vi "PECT - Scan no trigger.vi"() -> ()   [LabVIEW 2018]
uses:
  <vilib>/DAQmx/write.llb/DAQmx Write (Analog 1D Wfm NChan NSamp).vi
  <vilib>/DAQmx/read.llb/DAQmx Read (Analog 1D DBL 1Chan NSamp).vi
  <vilib>/DAQmx/read.llb/DAQmx Read (Analog Wfm 1Chan NSamp).vi
  <vilib>/DAQmx/create/channels.llb/DAQmx Create Channel (AI-Voltage-Basic).vi
  <vilib>/DAQmx/configure/timing.llb/DAQmx Timing (Sample Clock).vi
  <vilib>/DAQmx/configure/task.llb/DAQmx Configure Logging (TDMS).vi
  <vilib>/DAQmx/configure/trigger.llb/DAQmx Start Trigger (Digital Edge).vi
  <vilib>/DAQmx/create/channels.llb/DAQmx Create Channel (AO-Voltage-Basic).vi
  <vilib>/DAQmx/miscellaneous.llb/DAQmx Fill In Error Info.vi
  <vilib>/Instr/_visa.llb/VISA Configure Serial Port (Instr).vi
  <vilib>/express/express analysis/Spectral/Block/exnSpectralBlock spectral measurements PSD poly.vi
  <vilib>/express/express analysis/Spectral/Block/exnSpectralBlock spectral measurements PSD WFM.vi
  <vilib>/express/express analysis/Spectral/XNode/ExpressSpectralMeasurementsBlockNode.xnode
  <resource>/objmgr/daqmx.rc
  <vilib>/measure/NI_MABase.lvlib
  <vilib>/Platform/NI_3dgraph.lvlib
  <vilib>/DAQmx/read.llb/DAQmx Read (Counter U32 1Chan 1Samp).vi
  <vilib>/DAQmx/create/channels.llb/DAQmx Create Channel (CI-Count Edges).vi
panel:
  out "숫자형 2":i32
  out "숫자형 3":i32
  in  "Stop Scan 2":bool
  in  "Scan 2":bool caption="Scan"
  in  "Move Distance (mm)":dbl=16.64
  in  "Counter":tag="Dev1/ctr0"
  in  "ViewMode Analysis":i32(ring) items=["cwViewXYPlane", "cwViewXZPlane", "cwViewYZPlane", "cwViewUserDefined"]
  in  "Plot style Analysis":i32(ring)=5 items=["cwLine"=1, "cwPoint"=2, "cwLinePoint"=3, "cwHiddenLine"=4, "cwSurface"=5, "cwSurfaceLine"=6, "cwSurfaceNormal"=7, "cwContourLine"=8, "cwSurfaceContour"=9]
  in  "Open":bool
  in  "Save Scan mode":bool caption="Save Process"
  in  "Tab Control 2":T1(tab)
  out "Hall sensors signal":waveform(dbl)[](graph)=[{"t0"=timestamp(3525645621.636764 s since 1904-01-01), "dt"=1.9999999999999944e-06, "Y"=array[2100 elements], "attributes"=variant("NI_ChannelName"=variant(string "Dev1/ai0"), "NI_UnitDescription"=variant(string "Volts"))}, {"t0"=timestamp(3525645621.636764 s since 1904-01-01), "dt"=1.9999999999999944e-06, "Y"=array[2100 elements], "attributes"=variant("NI_ChannelName"=variant(string "Dev1/ai0"), "NI_UnitDescription"=variant(string "Volts"))}]
  out "Feature Extraction":dbl(graph)=0.021153968958947764
  out "Waveform Graph 2":waveform(dbl)[](graph)=[{"t0"=timestamp(0 s since 1904-01-01), "dt"=1.25e-06, "Y"=array[8000 elements]}]
  out "Power spectral density":cluster{"f0":dbl, "df":dbl, "magnitude":dbl[]}[](graph)=[{"f0"=0.0, "df"=238.09523809523876, "magnitude"=[-25.4340272409559, -28.495970805276507, -69.09064054555873, -79.11355871279994, -75.69366097931027, -84.18131507822396, -80.50168881348966, -82.72314293089615, -87.19630499623688, -82.83568021481967, -89.95290866002237, -85.90392585035596, -87.41269111550386, -91.40893948681482, -86.69370819914215, -93.36336146616782, -89.019380476413, -89.73232030153878, -94.58261196624535, -89.16287927388944, -94.965890302584, -91.86846413178648, -91.95327957161693, -97.62687167891286, -91.59993648735762, -97.30685711015555, -93.8350762480425, -93.27921214218685, -99.59438563802183, -93.1824258709588, -98.3113125531512, -95.45425138584356, -94.39327135467576, -100.65352961491782, -94.55889081970952, -99.40788907105079, -97.93617495318924, -96.19517579047603, -103.97036797797732, -96.40295202889732, -99.7036956909043, -99.48760137175819, -97.46192979187015, -106.29271483151813, -97.51447379981207, -99.86179280251669, -100.43811038443037, -97.59011642740829, -105.58363666166275, -99.01126121197593, -101.01575323613292, -101.90167607549864, -98.61952569586691, -106.73670466995647, -99.29976101634999, -101.54959604687718, -105.17330050767885, -100.09392305285375, -109.78264848704497, -100.98914236173123, -101.81665207962125, -105.42358374403365, -99.82880728595141, -107.07330885402075, -101.07712607444097, -101.03780825357597, -107.32811151840846, -101.221643458408, -105.63776326231454, -101.8420593566944, -101.80081629073969, -107.47915505307212, -101.12986632760553, -106.84901404755908, -102.73715610491038, -101.51552854007832, -107.28771371003282, -101.3928633472346, -107.44515355816633, -104.89304864643535, -103.1455098860718, -110.19910428997925, -102.73063833081197, -107.57101838377707, -104.90574568581201, -103.72599931018533, -109.97178587260123, -103.24611921258705, -108.36098023558972, -106.6408311450923, -104.73569536588386, -116.21683530762306, -105.02627439976544, -107.15856030450797, -109.81191038702062, -105.53476822084077, -119.10077766590356, -105.31867536160968, -106.9718410299748, -108.34458911268797, -104.70307996109247, -114.76704583683203, -106.29948298493936, -108.55077108437321, -112.16618350190343, -105.98453547558171, -114.68576835450673, -107.50968901677987, -107.89174277914348, -111.59875709602721, -106.69368240333122, -114.93273233954758, -105.23904516482949, -106.00272331017348, -110.36103151258544, -104.93177986717492, -110.8835476773746, -106.69346348818806, -106.66103973993782, -119.11729839814336, -108.06338160849775, -114.5879267769655, -108.59816838472844, -107.53189260743514, -114.07390818184973, -106.70996756049796, -113.27381274118753, -109.50270539577696, -107.37282420343303, -113.4779718725949, -106.04267666963091, -111.30294425571472, -112.46717993668915, -109.13164915488709, -116.65287200885172, -107.03002573045511, -110.21479040603631, -112.476075561056, -106.97710947409149, -119.42145279296255, -108.3200486628316, -110.46641858585929, -117.16650627564961, -109.73297826697552, -120.31689830731365, -107.19513745371916, -110.66663569403087, -113.30365980039964, -110.01971553524372, -123.68660617105166, -110.8171755739396, -111.11382172813546, -117.76239209582961, -109.49899370205401, -115.22252846498625, -111.1932077339224, -112.38235939086871, -118.22207022901702, -110.6546796895719, -116.97450780644367, -110.82401674194465, -111.96705198878843, -118.28092956599232, -110.5621503678909, -121.25720613496851, -111.98371482341479, -113.27928013246557, -111.96833712758355, -108.56859286664552, -120.32790468431601, -110.82699792221703, -110.79062667340345, -122.65756767769517, -110.48843456045427, -116.8782055296399, -115.43719816168479, -114.47619780315773, -121.42183196132746, -111.60631415727042, -120.68077308056417, -109.35478690141552, -109.03210709352732, -120.6260555904793, -109.47936424950136, -113.33719701518146, -112.88325992990137, -110.99901978536154, -123.19636626521421, -109.09861317900774, -113.33125158106256, -115.35673297389727, -112.77249677632989, -124.61163141716472, -114.68140920359865, -121.89642913325117, -115.47413298424323, -112.82196063671608, -127.87542521315149, -111.54178118788309, -113.6448752704395, -120.76569423868874, -112.98651214877823, -123.18868565400437, -115.41399838634062, -115.46853076016815, -116.40989072804102, -110.69611347288615, -132.23164080331392, -114.76376391429793, -121.7246597336247, -117.46893009589195, -114.01899156779395, -125.22079066032327, -114.59524199183258, -114.50034890537415, -122.9532092227648, -113.72727798159212, -125.65163915514907, -113.4793801211504, -110.4090756414644, -125.63592649005872, -114.22938378193007, -116.74947251106808, -121.60535557984142, -116.79385283402802, -122.44667696630361, -113.43873413563811, -123.28159708694415, -113.92892974938164, -114.01193823589753, -121.62751955742443, -118.76839573694522, -125.52998605097204, -115.19609643487229, -117.49409595176479, -117.08423885198002, -119.48314867245172, -125.01675515413412, -117.92668164142911, -115.55962389856793, -125.63488616674975, -119.11862859365166, -114.78860770332909, -117.18339781294443, -111.18063004722558, -118.31775966044624, -111.6867367949252, -114.57226159377, -119.36541212960576, -113.90245139442648, -132.46343443313128, -120.1282759002165, -121.05279009698619, -118.9115822659523, -121.23280439248342, -116.31914159559688, -127.38829313950257, -117.34673005740623, -115.95249861902771, -114.9301657394146, -123.22361802797445, -110.83274939062106, -116.16624248562111, -116.76753364192771, -113.94454545069023, -122.95736945775944, -118.66755800656253, -129.1462641201204, -116.6351050110328, -117.22529407303742, -123.80212197360244, -115.89792176423389, -114.25823938606595, -125.60467961977515, -114.59958849364433, -121.70071005514421, -118.25968972451209, -114.69929400946009, -123.88209034116528, -115.03869272537257, -117.52034211782204, -115.27990843516797, -117.85366603932033, -125.16865559622727, -118.21960424638507, -119.69008755413566, -117.24640963460672, -114.32867295013791, -119.1576982419508, -122.85495988425586, -116.3373010103401, -114.53730203699834, -115.67017599990201, -127.144321037601, -115.73849102686786, -117.7626163106355, -119.7346592991025, -117.41317517684553, -125.0417974461613, -114.5488949833583, -116.59812516173781, -119.91064563147799, -115.27933218667663, -122.09990513751134, -120.95678574143693, -123.25641714743752, -112.5173710452192, -113.53735878806998, -129.23914933506734, -116.27157269711533, -148.4020512032711, -118.84888216023774, -123.82550527215588, -116.87770979616658, -111.32191810025745, -124.32675905891588, -114.37182733794062, -121.10713785851372, -122.59698730059695, -116.38346694563282, -121.69144349152856, -119.00883142493832, -110.81886738196273, -120.7909830607913, -115.01780448665316, -114.52055121633796, -132.6824191654361, -116.330695115645, -126.4664151018508, -118.32717907779282, -118.7288071595281, -120.42749846140066, -112.53185615773879, -124.26026008984286, -114.24089252048742, -120.00368190003405, -114.71738500842926, -112.92262025927133, -129.21127897188563, -113.5947811765517, -117.80802009651353, -117.0133790103226, -112.19210322760304, -118.17549968071762, -119.3256187825503, -118.84981507334446, -121.39118969751144, -114.64543555194373, -119.84814933224528, -114.09123407848944, -116.22899352170892, -116.41650104077173, -113.70057202673476, -124.52773908304957, -114.87372641784933, -116.11651108221098, -121.68680962246994, -115.78306007961302, -122.22621008657796, -118.81157995182392, -113.9402115821658, -132.636729517989, -114.49554876936634, -119.50980190398928, -123.27410972236837, -118.52851881066383, -122.25212982572599, -117.13947036230024, -120.85005588797962, -118.41526503460501, -117.61788553858068, -126.3872056783977, -114.98198608543298, -119.7789938911847, -120.84873579392627, -114.38831474301695, -153.35954756825245, -113.19505610638078, -114.17454820985151, -127.41069917723112, -114.92677241657191, -125.49053973810628, -113.36382196587914, -119.96785250843519, -122.47388530423243, -116.38671253508838, -120.0905790211523, -119.83326265062107, -117.88168146696918, -122.3132169880757, -115.87324909105399, -125.92003267803432, -113.96860176867415, -114.49156118371398, -127.52634390035722, -115.05967156528004, -126.82020221981517, -117.93643187259194, -116.51163213641807, -119.47551219110167, -119.55225172256931, -116.9512257852571, -122.23153124485954, -120.8368476753637, -121.48473913072222, -115.83122660909913, -135.74260014140523, -116.58358375805423, -118.15236945484727, -119.06674062398864, -115.7844834762477, -125.06111738611818, -114.7801535050972, -115.2696605691888, -123.98656374010793, -119.29025555731172, -118.29146803784099, -119.55696172158135, -118.06884171238352, -127.81587648134607, -120.41730580797976, -123.49626136731604, -112.2147141798107, -116.22555232584983, -132.79419178871254, -119.66964883124663, -117.20946469243259, -118.20939292735417, -115.6951914646649, -129.64892855822356, -114.27056999288617, -120.31005512957381, -117.41846777372632, -115.50158386260813, -124.69777160737624, -115.2892897247205, -123.61522771666871, -113.75248734362687, -113.22999749252833, -129.3490509395313, -116.88137735661701, -116.94110280242681, -119.50244079984806, -119.30521139999144, -128.17199984115797, -118.06736594940236, -116.05331575995922, -121.29670750650897, -116.1140297602044, -125.090619084802, -121.41807296062154, -120.01332757902264, -120.54914530643151, -116.49738633175463, -122.32551291835904, -118.3190808346865, -118.92638453656723, -122.48819531011718, -117.01021725424317, -120.98896352560598, -117.23831688685218, -121.27915259197124, -121.20017251921661, -117.6155648860373, -120.91300272912063, -117.94438460863424, -115.94437430101533, -123.35904829443987, -117.74011174503076, -121.54935745388448, -120.82564553545025, -121.98951430455743, -120.24858103448778, -116.44403527138395, -112.79571494351876, -112.42801913096545, -110.1697573019791, -115.34500457736401, -119.81921052956707, -129.82600951154313, -115.5862301263047, -112.59292882433087, -120.79009137478283, -131.32849293387295, -113.61194478398238, -123.48568856527031, -119.17507777781304, -123.09261867490484, -116.97755217417308, -123.94453461434183, -116.58080525616379, -119.64289646280756, -122.90202645580743, -126.66219093058154, -121.95048829056148, -115.72578023509817, -116.70117814464484, -121.91050280869723, -118.25299095698178, -116.45905559047064, -132.57794493731578, -121.65327820443292, -120.9816664775787, -117.17270262269045, -120.27433984830965, -125.89418976028173, -119.09563505847817, -126.9693215534833, -113.17465524665704, -118.98702092883116, -119.83822568580342, -120.45832738089722, -120.67735960513633, -127.38676010839353, -127.65777338183055, -118.37446329057411, -115.61355494839711, -119.94568688114103, -116.06619937633681, -126.348857777089, -118.92850079147068, -119.5416617639739, -132.47075644221843, -118.08809356028496, -123.16186463092723, -121.51579486791232, -122.88983670053283, -129.5195538417256, -120.4730389608841, -132.16486858341602, -122.34690358436781, -120.71922104337597, -114.29260860841114, -117.67902631803368, -124.7040155514909, -123.51274592117205, -120.02297921674332, -136.54655493811157, -120.45629227407751, -119.06410204276258, -127.91681714792554, -122.82090055753153, -125.16838176650813, -121.79565386970478, -119.79607311590995, -126.54861375039647, -121.59135878113302, -132.8348640697562, -118.1305434733294, -120.46070148841905, -122.69571910896963, -117.6534954653865, -124.15742546824006, -120.73646926947502, -124.82696993800742, -124.513836786494, -123.15395713389651, -124.62395468806395, -117.21365768658171, -119.32635871968456, -121.48532284413152, -119.38242892643675, -126.25575652510352, -123.27133124029851, -117.58533922728374, -118.17710108929799, -114.99496360200965, -117.77133194647278, -111.34898201101595, -111.50817058307922, -119.0703124690998, -127.70676079885351, -121.8704969141074, -125.93154214283446, -118.65628450081473, -122.47918878348962, -117.9651589546518, -126.13560583004508, -122.42294805637847, -133.924453763793, -117.2082573038767, -117.6525335446734, -122.92077297426977, -122.04624645756786, -116.43289028226238, -117.93180959338378, -129.02356734231915, -117.95493621286326, -120.7555929766252, -120.76782849311112, -123.06287498470708, -117.83798593857965, -123.43423215434719, -120.15190119516652, -120.48240443128407, -143.29738987393452, -123.46572247444769, -120.89055325172792, -125.66715973809033, -118.26887578998644, -117.01836200028421, -121.33021830755509, -119.68846363313813, -122.60689066103069, -116.26858138914181, -119.59360791972998, -122.94866175463353, -114.174409515556, -118.00516930888391, -121.56978543579633, -135.87799017759036, -117.50816594504829, -122.82539428457626, -123.82103443155845, -124.77975840345442, -121.13340798086698, -120.93607435603558, -133.15787160745222, -120.70545628137863, -125.02155972441679, -122.04666465472178, -118.01234649746348, -127.88767491042842, -119.02096620167217, -120.16031065152875, -122.25406107859625, -121.72733059051095, -120.61357375519918, -118.63962847172827, -134.3857741605498, -116.3600853185034, -117.26695700691671, -119.9176982185873, -113.45576465218444, -126.69779573632724, -114.39554522802246, -116.8457146515868, -116.34219889483086, -119.30011291548334, -120.01163291843496, -114.29497178248809, -127.65687642749229, -119.58556923753022, -129.8593054181261, -122.2353645100479, -120.79536520223796, -119.83284028355028, -117.7991246185715, -128.390292904734, -119.78079925213122, -125.478913448993, -113.89747777944768, -112.66620124153357, -124.3475049842711, -120.85847303094337, -132.91807981902295, -119.523494985723, -116.65149909866443, -119.73287290436721, -127.63237851524192, -127.23413304048789, -120.87585453904362, -121.08540368080186, -134.91071939669257, -117.75375801669338, -117.2683014590723, -120.9739099492833, -118.23809733632451, -120.94065804928206, -123.88077510875804, -118.13812819300607, -122.60294123365466, -126.97075898006995, -120.18754789731035, -124.71238663441227, -120.55456557278582, -130.94599087480253, -111.18288669417035, -112.27708791831247, -126.0512034600378, -117.41881712783596, -128.20553880273903, -117.29482600885808, -118.2045526390752, -127.81966672699878, -117.03716165902529, -115.46711739757512, -117.15363929234843, -121.87599671671335, -121.19736800869221, -126.5301786755875, -131.20754947382918, -124.40138004810741, -129.0562496906515, -121.06816554587536, -121.01023627802867, -138.6137911215848, -120.12495002524031, -121.38510517514229, -122.79804220535513, -116.97501378195477, -118.82011581137473, -114.0229185604644, -119.54287501990726, -114.64474566771625, -117.76935669872461, -123.81082574158907, -118.51678358865587, -128.9664755188374, -123.45357998434133, -122.74888841574231, -120.74640581234044, -126.956344345126, -119.95682140104577, -118.8873101779055, -124.41062359284174, -128.97304498664363, -123.86287113204068, -127.30257087528216, -120.61364220528216, -114.45119129304715, -119.68384044686806, -131.29639185291157, -122.31250766293485, -119.57420865241102, -124.74014026002448, -124.87593035709094, -118.4566565612952, -123.76236085976001, -120.84780538841838, -117.68987599773281, -135.06195695255914, -122.56143585795171, -129.04610316842883, -118.32313199570537, -117.77093802786419, -124.46572845786741, -129.1123298336903, -120.88470269965448, -116.69988985752187, -116.84054667499878, -133.76883696987278, -122.32434984927302, -124.98940594457933, -122.56515592789917, -118.31562562243366, -133.97049179545627, -122.33220627999802, -131.16753675316977, -124.69828063969263, -116.37621154460467, -126.1833423168025, -129.62937634161355, -118.46241371150788, -117.52851478852457, -125.32425037236442, -119.0327364293772, -124.2861355894013, -123.24573502278234, -125.52155812053758, -113.75743410709823, -114.79513162658353, -128.58142362588052, -122.48277095196701, -118.94747544412269, -123.86988127835491, -124.78140456983323, -121.53998481875398, -116.01432822539552, -119.20174681160661, -122.75167725800814, -120.58657749420254, -118.51141061842183, -119.24457006171983, -131.43641234223372, -116.00759139055087, -121.24442216102587, -123.29371279953725, -117.608355420454, -116.33684374617326, -118.06291688281922, -121.88761866022774, -121.54820313120047, -119.5051369873635, -126.56611158390913, -118.84012713615805, -121.09285296522563, -124.67955377692547, -147.31451139022337, -116.80660421066897, -114.8367853755961, -120.41026468628925, -123.65666101895222, -119.64837119787269, -116.77480172559095, -116.54263359173909, -124.75286620868079, -117.33721912698883, -116.51795620907136, -118.50086748176733, -128.10381328920522, -122.78098994574157, -120.24716756092855, -119.52743204722819, -115.00407387659232, -108.2853711552629, -108.61086943894702, -119.6228894146785, -124.11132022420912, -125.6202218409766, -123.1749360787656, -118.1971196161698, -123.95075368058998, -121.72140109898365, -123.27106899042522, -123.73035629887062, -121.24369679109273, -121.07381526465288, -113.13965659723667, -118.330755475899, -118.40249076804484, -111.59630598649044, -116.1569506845575, -125.67326089915758, -125.85723567111906, -119.24293277595024, -117.87067617433537, -120.70936924059559, -131.8090588468898, -132.98711569625004, -123.63274249467587, -122.75476917502559, -126.12873814250243, -120.53144270605179, -129.07030822919336, -122.7889410422919, -124.35405971166259, -119.63968579420454, -139.0154441054289, -129.47962001806934, -121.86548015410847, -128.6818469257012, -121.40195873232601, -138.64231053781285, -124.22025721762265, -124.06073958736941, -126.71929802352521, -131.7498459276443, -120.68144109742178, -122.6325588818875, -126.80796617875095, -124.92487955227033, -136.94498040498806, -124.26704334219014, -123.21376211221711, -140.25352033075964, -129.53222319772195, -122.58541579060463, -122.1996729592375, -125.66642108013673, -125.66310429236694, -120.09682773706965, -125.27326633941439, -121.55721878725502, -121.22507119941083, -121.53716878624485, -136.20685498111987, -128.15260146013156, -120.03473972471616, -124.60755958763912, -124.73082500077143, -123.93425949983688, -131.04483249265184, -121.7957035014449, -127.09321441816094, -133.6144579272493, -124.69014595896968, -130.4902091211609, -121.18031440773905, -128.00033943961677, -125.88991118115149, -118.865310745079, -123.69668867733147, -117.98756965862728, -114.40013091842827, -118.28685032521078, -122.23464196869948, -124.8440422629961, -129.66281606870848, -119.440534215621, -124.54391783563877, -124.93447967158188, -121.7258558761523, -122.28817885403082, -127.06889620458577, -128.92172974939206, -120.62932166634072, -126.06847321900452, -123.31471168429935, -121.80350826545656, -129.2574604322076, -125.67225933193998, -125.7801671825605, -129.53804733161627, -119.56756644124712, -128.82490314699373, -124.7689736295626, -120.50019729114693, -124.50603158563972, -122.8120627011088, -125.60528875555717, -123.8817354922713, -124.05570537836674, -120.94568834491936, -118.06056028605255, -124.24390361274648, -125.5716703018188, -127.71949519914061, -130.7001652968252, -126.27701412017494, -133.76810134709916, -128.4738939614179, -120.302550881701, -118.91298143662928, -124.9077318110765, -127.16253699189492, -118.11405934812818, -117.52028071290711, -140.95620572748925, -123.61977932545628, -131.0334379970501, -125.88948384968432, -127.81552331993379, -121.92316280719056, -119.05911238768732, -126.83773251459189, -123.52627415002164, -120.8779561023192, -123.66683567603742, -131.64300993967345, -123.62895847772963, -116.89792951363142, -120.1068259250195, -117.92484706459337, -115.58208487778379, -120.76803581628594, -123.95408562090736, -122.79456549632754, -134.5305398779298, -123.57040300991032, -128.40634159414552, -123.70102187824159, -118.24970739397313, -119.66483900349026, -127.78024313111393, -120.3547204111785, -125.49305364308705, -119.49505591004302, -120.50920386196539, -119.03509516851003, -114.24667300009652, -121.60538636584391, -119.95304417598024, -122.24585853682832, -128.63653016912684, -116.04810628805795, -121.94159862131235, -122.59928204398939, -121.4532410501923, -128.6511474663462, -130.83715595958148, -121.71998300574741, -116.91426629511156, -113.587592058512, -115.59736707638731, -124.65300822631244, -133.32538684258748, -124.02289142873636, -121.54278890993639, -119.02596809402394, -108.90572887117857, -112.14974069608851, -129.21149299565423, -118.82148342951197, -116.65510894288538, -118.39609618084175, -116.53502642884725, -122.47549439965209, -122.23125657046063, -123.68081343116663, -120.67915071600007, -123.6899360128769, -118.56721985209728, -118.36641581191942, -126.96724630704657, -119.36877661672403, -123.07698921198843, -117.80772421906035, -122.82545076270567, -118.82755071380888, -117.21030132539394, -129.760567864525, -118.0816708063509, -125.80573274113647, -121.18434666182338, -121.80987210832065, -130.99259828357094, -125.47223579895922, -123.86818606677002, -118.7118158196511, -119.27778317338742, -127.27333258839096, -119.90672352079164, -140.78772370844268, -118.08251080057329, -119.86636232122572, -118.69482489738232, -119.19106512767372, -123.70988914879189, -121.92566832147995, -123.41378261726373, -120.1715186070818, -117.9079629421116, -117.41960207545632, -123.72833996166874, -127.24377206607298, -124.99098647980887, -129.48803701799955, -129.92351350561592, -120.79284154834647, -119.29601975194524, -136.17244775530037, -126.73975437546255, -128.84068276143336, -125.66374985701982, -136.69026010435715, -125.44409235146617, -119.28138070315057, -118.65017329869724, -118.02521532826772, -122.23736063759657, -121.27846943548622, -116.69850478126861, -119.7711336696722, -123.70776561180185, -118.43344549561263, -123.92390877157247, -117.19637143066551, -117.64112988205311, -127.78399195238529]}, ...(2 in all)]
  in  "3D Surface":refnum<k7>(container)
  out "Feature Extraction 2":dbl(graph)=0.021153968958947764
  in  "Emergency Stop":bool
  in  "Stop 3":bool
  in  "Home Y":bool
  in  "Home X":bool
  in  "Back":bool
  in  "Front":bool
  in  "Left":bool
  in  "Right":bool
  in  "Stop Scan":bool
  in  "Scan":bool
  in  "Tab Control":enum32{"     Motor    ", "         DAQ        "}(tab)
  out "Y line":i32 caption="Y percent"
  in  "Move X":bool
  in  "X-length":dbl=20.0
  in  "Y-length":dbl=20.0
  in  "Step Y":dbl=0.2
  in  "1 Min":dbl=0.4
  in  "2 Max":dbl=6.0
  in  "1  Max":dbl=6.0
  in  "2 Min":dbl=0.4
  in  "1 Rate":dbl=0.2
  in  "2 Rate":dbl=0.4
  in  "Travel per Pulse (mm)":dbl=0.002
  in  "Cur. Pos X":dbl=-33.28 format="%#.4f"
  in  "Cur. Pos Y":dbl=30.0 format="%#.4f"
  in  "Save Speed":bool
  in  "COM Port":refnum<visa-resource-name>="COM4"
  in  "Baud Rate":u32=9600
  in  "Data bits":u16=8 min=5 max=8 step=1
  in  "stop bits":u16(ring)=10 items=["1.0"=10, "1.5"=15, "2.0"=20]
  in  "Parity":u16(ring) items=["None", "Odd", "Even", "Mark", "Space"]
  in  "Logging Mode":i32(ring)=10231 items=["Off"=10231, "Log and Read"=15842]
  out "Actual Sample Rate":dbl=500000.0 format="%0.2f"
  in  "Physical Channel":tag="Dev4/ai0"
  in  "Min Voltage":dbl=-10.0
  in  "Max Voltage":dbl=10.0
  in  "Terminal Configuration":i32(ring)=10083 items=["default"=-1, "RSE"=10083, "NRSE"=10078, "Differential"=10106, "Pseudodifferential"=12529]
  in  "Sample Clock Source 2":tag="OnboardClock"
  in  "Sample Rate":dbl=500000.0
  in  "TDMS File Path":path
  in  "Number of Samples 2":i32=160
  out "Actual Sample Rate 2":dbl=800000.0 format="%0.2f"
  in  "Physical Channel(s)":tag="Dev4/ao1"
  in  "Min Voltage 2":dbl=-10.0
  in  "Max Voltage 2":dbl=10.0
  in  "Sample Clock Source":tag="OnboardClock"
  in  "Sample Rate 2":dbl=800000.0
  in  "Number of Samples":i32=8000
  in  "Offset":bool
  in  "2 Plots":bool
  in  "Edge":i32(ring)=10280 items=["Rising"=10280, "Falling"=10171]
  in  "Digital Trigger Source":tag="/Dev4/PFI0"
  in  "Average":i32=10
  in  "Duty cycle %":dbl=50.0 format="%#.2f"
  in  "Stop":bool
  in  "Output Array":T2(array[cluster])=[{"Waveform Type"=2, "Amplitude"=10.0, "Frequency"=300.0}] {"Frequency" format="%0.2p"; "Amplitude" format="%0.2p"; "Waveform Type" items=["Sine Wave", "Triangle Wave", "Square Wave", "Sawtooth Wave"]}
  # "Pulse Shape"
  # "Trigger Settings"
  # "Data Processing"
  # "Pulse"
  # "Hall Sensors Signal"
  # "Feature Extraction"
  # "Power Spectal Density"
  # "COM  Setting"
  # "Speed  Setting"
  # "Scan  Setting"
  # "Pulse  Channel"
  # "Pulse  Timming"
  # "Sensor  Channel"
  # "DAQ Timming"
  # "Logging Settings"
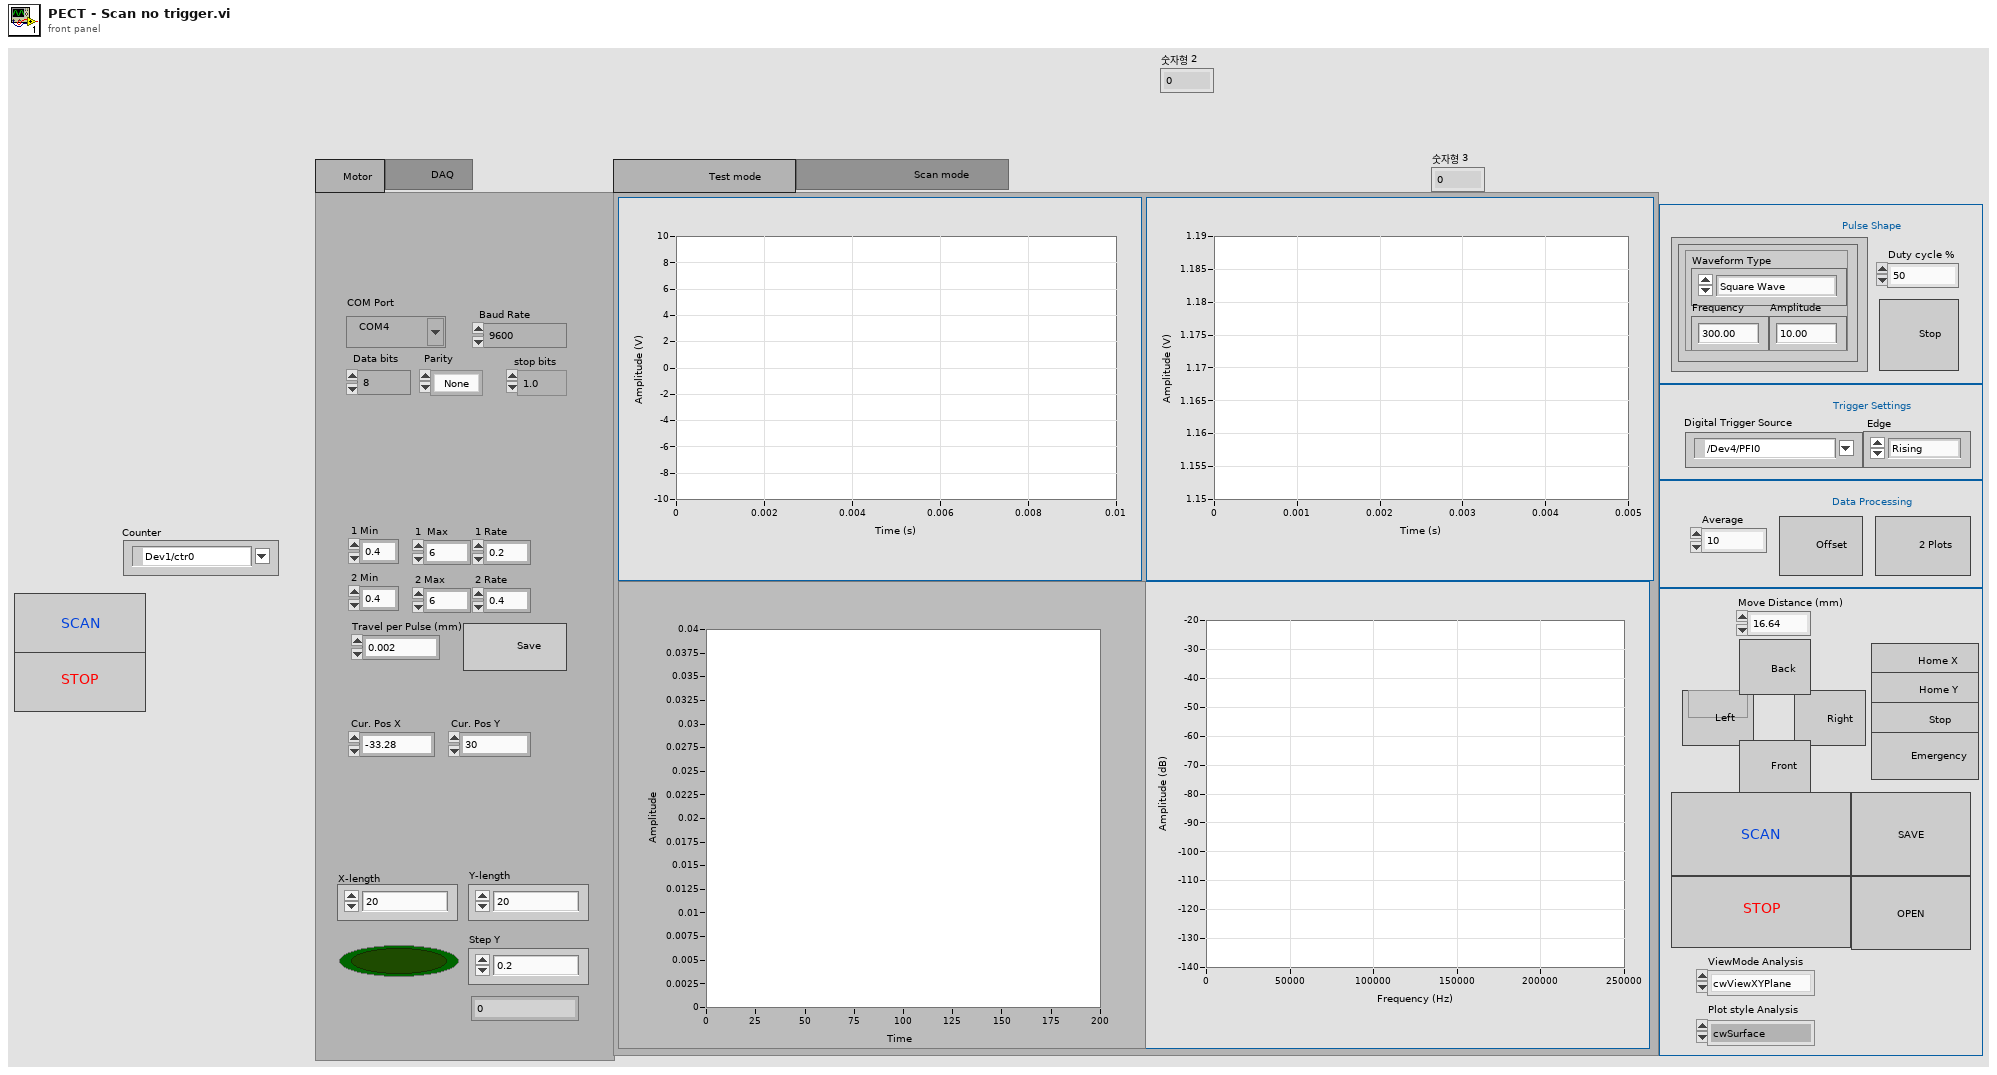
[diagram p1: front panel]
types:
  T1 = enum32{"                    Test mode                   ", "                          Scan mode                      "}
  T2 = cluster{"Waveform Type":u16, "Amplitude":dbl, "Frequency":dbl}[]
  T3 = cluster{"Waveform Type":u16, "Amplitude":dbl, "Frequency":dbl}
  T4 = cluster{"averaging mode":u16, "weighting mode":u16, "number of averages":u32}
  T5 = cluster{"dB On (F)":bool, "unwrap phase (F)":bool, "convert to degree (F)":bool}
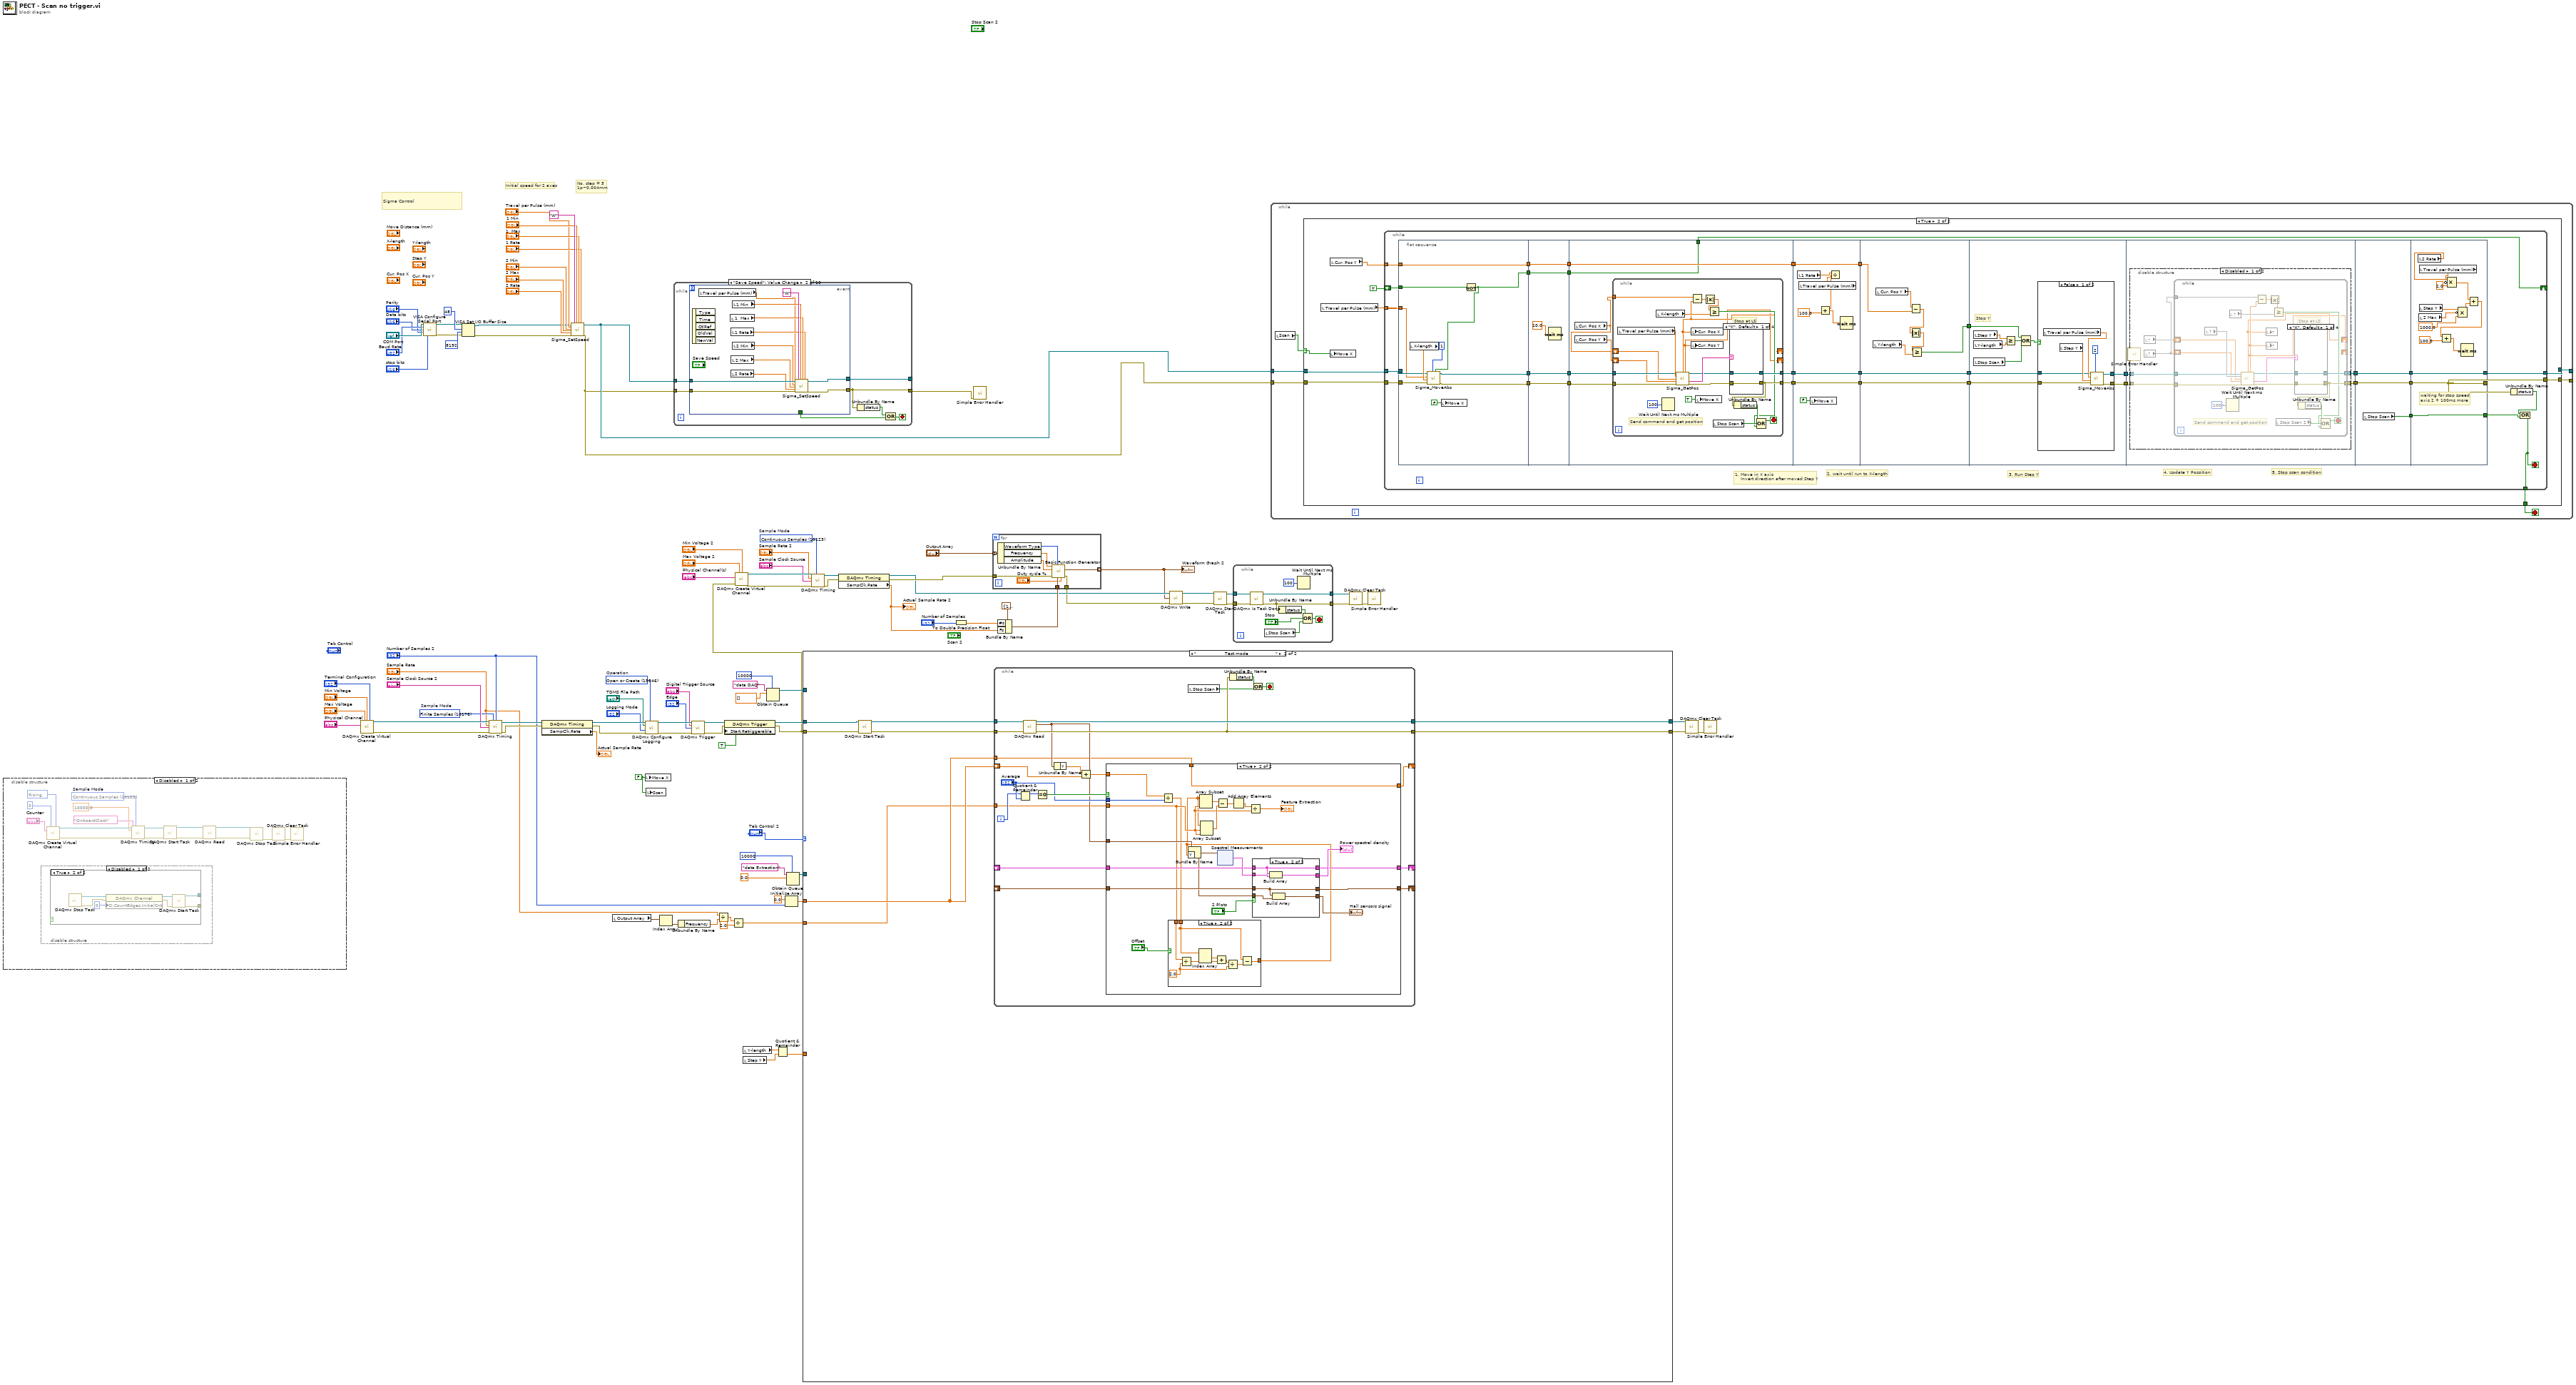
[diagram p0: block diagram]
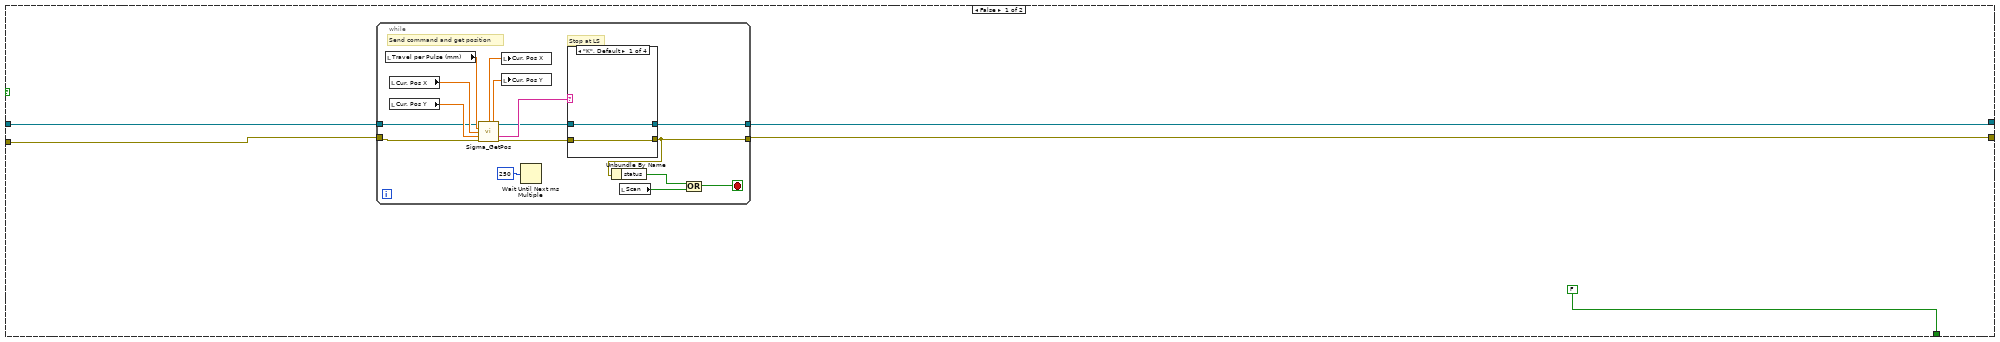
[diagram p2: hidden frame]
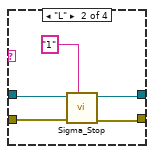
[diagram p3: hidden frame]
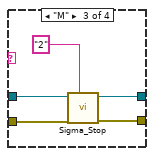
[diagram p4: hidden frame]
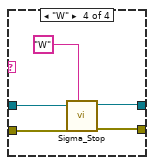
[diagram p5: hidden frame]
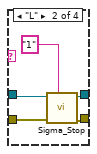
[diagram p6: hidden frame]
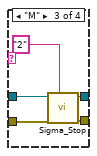
[diagram p7: hidden frame]
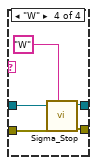
[diagram p8: hidden frame]
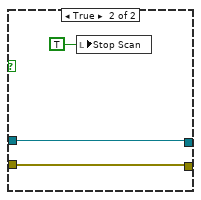
[diagram p9: hidden frame]
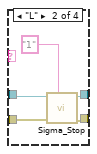
[diagram p10: hidden frame]
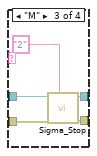
[diagram p11: hidden frame]
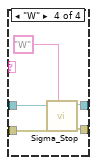
[diagram p12: hidden frame]
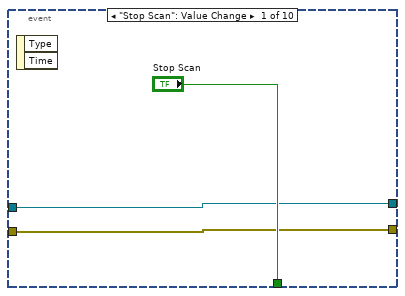
[diagram p14: hidden frame]
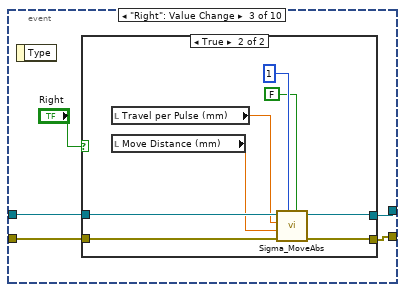
[diagram p15: hidden frame]
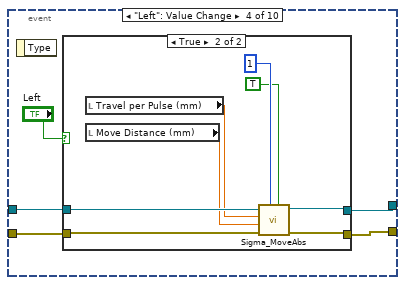
[diagram p17: hidden frame]
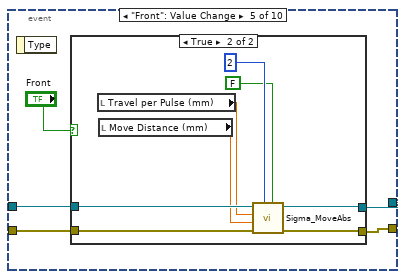
[diagram p19: hidden frame]
diagram:
  w1 = FALSE ("Move X")
  w55 = 10178 items=["Finite Samples"=10178, "Continuous Samples"=10123, "Hardware Timed Single Point"=12522]  # Sample Mode
  w78 = 10123 items=["Finite Samples"=10178, "Continuous Samples"=10123, "Hardware Timed Single Point"=12522]  # Sample Mode
  w94 = 15846 items=["Open"=10437, "Open or Create"=15846, "Create or Replace"=15847, "Create"=15848]  # Operation
  # "No. step = 5\n1p~0.004mm"
  # "Initial speed for 2 axes"
  # "Sigma Control"
  n1 = disable-structure shown="Disabled" {
    frame Disabled {
      w115 = 10280 items=["Rising"=10280, "Falling"=10171] ("edge")
      w114 = 10123 items=["Finite Samples"=10178, "Continuous Samples"=10123, "Hardware Timed Single Point"=12522]  # Sample Mode
      n2 = disable-structure shown="Disabled" {
        frame Disabled {
          n3 = case shown="True" {
            selector: _ -> [_ _]
            tunnel: [_ w120] -> _
            tunnel: [_ w117] -> _
            frame False {
            }
            frame True {
              n4 = call <vilib>:"DAQmx Stop Task.vi"() -> ("task out"=w122:refnum<k21>, "error out"=w119:errorcluster)  [unwired: 14 in]
              n5 = property class="DAQmx Channel"(reference=w122, error in=w119, "CI.CountEdges.InitialCnt"=u32 0) -> (reference out=w121:refnum<k21>, error out=w118:errorcluster)
              n6 = call <vilib>:"DAQmx Start Task.vi"("task/channels in"=w121, "error in"=w118) -> ("task out"=w120:refnum<k21>, "error out"=w117:errorcluster)  [unwired: 12 in]
            }
          }
        }
        frame Enabled {
        }
      }
      n7 = call-poly <vilib>:"DAQmx Create Virtual Channel.vi"("initial count"=u32 0, "edge"=w115, "counter"="Counter") -> ("task out"=w110:refnum<k21>, "error out"=w109:errorcluster)  [unwired: 11 in]
      n8 = call-poly <vilib>:"DAQmx Timing.vi"("task/channels in"=w110, "sample mode"=w114, "rate"=10000.0, "source"=tag "OnboardClock", "error in"=w109) -> ("task out"=w112:refnum<k21>, "error out"=w111:errorcluster)  [unwired: 9 in]
      n9 = call <vilib>:"DAQmx Start Task.vi"("task/channels in"=w112, "error in"=w111) -> ("task out"=w104:refnum<k21>, "error out"=w102:errorcluster)  [unwired: 12 in]
      n10 = call-poly <vilib>:"DAQmx Read.vi"("task/channels in"=w104, "error in"=w102) -> ("task out"=w103:refnum<k21>, "error out"=w101:errorcluster)  [unwired: 11 in, 1 out]
      n11 = call <vilib>:"DAQmx Stop Task.vi"("task/channels in"=w103, "error in"=w101) -> ("error out"=w106:errorcluster)  [unwired: 12 in, 1 out]
      n12 = call <vilib>:"DAQmx Clear Task.vi"("error in"=w106) -> ("error out"=w105:errorcluster)  [unwired: 14 in]
      n13 = call <vilib>:"Simple Error Handler.vi"("error in (no error)"=w105) -> ()  [unwired: 4 in, 5 out]
    }
    frame Enabled {
    }
  }
  n14 = call-poly <vilib>:"DAQmx Create Virtual Channel.vi"("maximum value"="Max Voltage", "minimum value"="Min Voltage", "input terminal configuration"="Terminal Configuration", "physical channels"="Physical Channel") -> ("task out"=w97:refnum<k21>, "error out"=w98:errorcluster)  [unwired: 10 in]
  n15 = call-poly "VISA Configure Serial Port"("VISA resource name"="COM Port", "baud rate (9600)"="Baud Rate", "data bits (8)"="Data bits", "parity (0:none)"="Parity", "stop bits (10: 1 bit)"="stop bits") -> ("VISA resource name out"=w12:refnum<visa-resource-name>, "error out"=w6:errorcluster)  [unwired: 9 in]
  n16 = VISA Set I/O Buffer Size(VISA resource name=w12, mask (16)=48, size (4096)=u32 8192, error in (no error)=w6) -> (VISA resource name out=w16:refnum<visa-resource-name>, error out=w15:errorcluster)
  n17 = call-poly <vilib>:"DAQmx Timing.vi"("task/channels in"=w97, "sample mode"=w55, "samples per channel"="Number of Samples 2", "rate"="Sample Rate", "source"="Sample Clock Source 2", "error in"=w98) -> ("task out"=w100:refnum<k21>, "error out"=w99:errorcluster)  [unwired: 8 in]
  n18 = property class="DAQmx Timing"(reference=w100, error in=w99) -> (reference out=w96:refnum<k21>, error out=w95:errorcluster, "SampClk.Rate"=→"Actual Sample Rate":dbl)
  n19 = call "Sigma_SetSpeed.vi"("VISA resource name"=w16, "Travel per Pulse (0.004mm)"="Travel per Pulse (mm)", "Min (1mm) 2"="2 Min", "Max (2mm) 2"="2 Max", "Rate (1mm) 2"="2 Rate", "error in (no error)"=w15, "Axis (1)"="W", "Min (1mm)"="1 Min", "Max (2mm)"="1  Max", "Rate (1mm)"="1 Rate") -> ("VISA resource name out"=w5:refnum<visa-resource-name>, "error out"=w4:errorcluster)  [unwired: 8 in]
  n20 = local read "Output Array"() -> (w45:T2)
  n21 = local write "Move X"(w1) -> ()
  n22 = call-poly <vilib>:"DAQmx Configure Logging.vi"("task/channels in"=w96, "operation"=w94, "file path"="TDMS File Path", "logging mode"="Logging Mode", "error in"=w95) -> ("task out"=w93:refnum<k21>, "error out"=w92:errorcluster)  [unwired: 9 in]
  n23 = local write "Scan"(w1) -> ()
  n24 = Index Array(array=w45) -> (element=w44:T3)  [unwired: 1 in]
  n25 = while {
    tunnel: w5 -> [w130]
    tunnel: [w125] -> _
    tunnel: w4 -> [w129]
    tunnel: [w127] -> w25
    stop <- w126 stop-if-true
    n26 = event shown="[1] \"Save Speed\": Value Change" {
      selector: _ -> [_ _ _ _ _ _ _ _ _ _]
      dyn-events: _ -> [_ _ _ _ _ _ _ _ _ _]
      timeout: _ -> [_ _ _ _ _ _ _ _ _ _]
      tunnel: w130 -> [w132 w145 w148 w163 w178 w193 w210 w222 w232 w244]
      tunnel: w129 -> [w131 w142 w147 w162 w177 w192 w209 w221 w231 w243]
      tunnel: [w132 w144 w150 w165 w180 w195 w207 w220 w234 w246] -> w125
      tunnel: [w131 w143 w149 w164 w179 w194 w206 w219 w233 w245] -> w127
      tunnel: ["Stop Scan" _ _ _ _ _ _ _ _ _] -> w124
      event "Stop Scan": Value Change {
        n27 = event-data() -> ()  [unwired: 1 in, 2 out]
      }
      event "Save Speed": Value Change {
        n28 = event-data() -> ()  [unwired: 1 in, 5 out]
        n29 = local read "Travel per Pulse (mm)"() -> (w134:dbl)
        n30 = local read "1  Max"() -> (w139:dbl)
        n31 = local read "1 Rate"() -> (w138:dbl)
        n32 = local read "2 Rate"() -> (w135:dbl)
        n33 = local read "2 Max"() -> (w136:dbl)
        n34 = local read "1 Min"() -> (w140:dbl)
        n35 = local read "2 Min"() -> (w137:dbl)
        n36 = call "Sigma_SetSpeed.vi"("VISA resource name"=w145, "Travel per Pulse (0.004mm)"=w134, "Min (1mm) 2"=w137, "Max (2mm) 2"=w136, "Rate (1mm) 2"=w135, "error in (no error)"=w142, "Axis (1)"="W", "Min (1mm)"=w140, "Max (2mm)"=w139, "Rate (1mm)"=w138) -> ("VISA resource name out"=w144:refnum<visa-resource-name>, "error out"=w143:errorcluster)  [unwired: 8 in]
      }
      event "Right": Value Change {
        n37 = event-data() -> ()  [unwired: 1 in, 1 out]
        n38 = case shown="True" "Right" {
          tunnel: [w152 w158] -> w150
          tunnel: [w151 w157] -> w149
          tunnel: w148 -> [w152 w160]
          tunnel: w147 -> [w151 w159]
          frame False {
          }
          frame True {
            n39 = local read "Travel per Pulse (mm)"() -> (w154:dbl)
            n40 = local read "Move Distance (mm)"() -> (w153:dbl)
            n41 = call "Sigma_MoveAbs.vi"("Direction (+)"=FALSE, "Axis (1)"=1, "error in (no error)"=w159, "Travel (1mm)"=w153, "Travel per Pulse (0.004mm)"=w154, "VISA resource name"=w160) -> ("error out"=w157:errorcluster, "VISA resource name out"=w158:refnum<visa-resource-name>)  [unwired: 4 in]
          }
        }
      }
      event "Left": Value Change {
        n42 = event-data() -> ()  [unwired: 1 in, 1 out]
        n43 = case shown="True" "Left" {
          tunnel: [w167 w174] -> w165
          tunnel: [w166 w173] -> w164
          tunnel: w163 -> [w167 w175]
          tunnel: w162 -> [w166 w172]
          frame False {
          }
          frame True {
            n44 = local read "Travel per Pulse (mm)"() -> (w169:dbl)
            n45 = local read "Move Distance (mm)"() -> (w168:dbl)
            n46 = call "Sigma_MoveAbs.vi"("Direction (+)"=TRUE, "Axis (1)"=1, "error in (no error)"=w172, "Travel (1mm)"=w168, "Travel per Pulse (0.004mm)"=w169, "VISA resource name"=w175) -> ("error out"=w173:errorcluster, "VISA resource name out"=w174:refnum<visa-resource-name>)  [unwired: 4 in]
          }
        }
      }
      event "Front": Value Change {
        n47 = event-data() -> ()  [unwired: 1 in, 1 out]
        n48 = case shown="True" "Front" {
          tunnel: [w182 w188] -> w180
          tunnel: [w181 w187] -> w179
          tunnel: w178 -> [w182 w190]
          tunnel: w177 -> [w181 w189]
          frame False {
          }
          frame True {
            n49 = local read "Travel per Pulse (mm)"() -> (w184:dbl)
            n50 = local read "Move Distance (mm)"() -> (w183:dbl)
            n51 = call "Sigma_MoveAbs.vi"("Direction (+)"=FALSE, "Axis (1)"=2, "error in (no error)"=w189, "Travel (1mm)"=w183, "Travel per Pulse (0.004mm)"=w184, "VISA resource name"=w190) -> ("error out"=w187:errorcluster, "VISA resource name out"=w188:refnum<visa-resource-name>)  [unwired: 4 in]
          }
        }
      }
      event "Back": Value Change {
        n52 = event-data() -> ()  [unwired: 1 in, 1 out]
        n53 = case shown="True" "Back" {
          tunnel: [w197 w203] -> w195
          tunnel: [w196 w202] -> w194
          tunnel: w193 -> [w197 w205]
          tunnel: w192 -> [w196 w204]
          frame False {
          }
          frame True {
            n54 = local read "Travel per Pulse (mm)"() -> (w199:dbl)
            n55 = local read "Move Distance (mm)"() -> (w198:dbl)
            n56 = call "Sigma_MoveAbs.vi"("Direction (+)"=TRUE, "Axis (1)"=2, "error in (no error)"=w204, "Travel (1mm)"=w198, "Travel per Pulse (0.004mm)"=w199, "VISA resource name"=w205) -> ("error out"=w202:errorcluster, "VISA resource name out"=w203:refnum<visa-resource-name>)  [unwired: 4 in]
          }
        }
      }
      event "Home X": Value Change {
        n57 = event-data() -> ()  [unwired: 1 in, 1 out]
        n58 = case shown="True" "Home X" {
          tunnel: [w212 w215] -> w207
          tunnel: [w211 w214] -> w206
          tunnel: w210 -> [w212 w217]
          tunnel: w209 -> [w211 w216]
          frame False {
          }
          frame True {
            n59 = call "Sigma_Home.vi"("Axis (1)"="1", "error in (no error)"=w216, "VISA resource name"=w217) -> ("error out"=w214:errorcluster, "VISA resource name out"=w215:refnum<visa-resource-name>)  [unwired: 7 in]
          }
        }
      }
      event "Home Y": Value Change {
        n60 = event-data() -> ()  [unwired: 1 in, 1 out]
        n61 = case shown="True" "Home Y" {
          tunnel: [w224 w227] -> w220
          tunnel: [w223 w226] -> w219
          tunnel: w222 -> [w224 w229]
          tunnel: w221 -> [w223 w228]
          frame False {
          }
          frame True {
            n62 = call "Sigma_Home.vi"("Axis (1)"="2", "error in (no error)"=w228, "VISA resource name"=w229) -> ("error out"=w226:errorcluster, "VISA resource name out"=w227:refnum<visa-resource-name>)  [unwired: 7 in]
          }
        }
      }
      event "Stop 3": Value Change {
        n63 = event-data() -> ()  [unwired: 1 in, 1 out]
        n64 = case shown="True" "Stop 3" {
          tunnel: [w236 w237] -> w234
          tunnel: [w235 w238] -> w233
          tunnel: w232 -> [w236 w240]
          tunnel: w231 -> [w235 w239]
          frame False {
          }
          frame True {
            n65 = call "Sigma_Stop.vi"("Axis (1)"="W", "error in (no error)"=w239, "VISA resource name"=w240) -> ("error out"=w238:errorcluster, "VISA resource name out"=w237:refnum<visa-resource-name>)  [unwired: 7 in]
          }
        }
      }
      event "Emergency Stop": Value Change {
        n66 = event-data() -> ()  [unwired: 1 in, 1 out]
        n67 = case shown="True" "Emergency Stop" {
          tunnel: [w248 w251] -> w246
          tunnel: [w247 w250] -> w245
          tunnel: w244 -> [w248 w253]
          tunnel: w243 -> [w247 w252]
          frame False {
          }
          frame True {
            n68 = call "Sigma_Stop.vi"("Axis (1)"="E", "error in (no error)"=w252, "VISA resource name"=w253) -> ("error out"=w250:errorcluster, "VISA resource name out"=w251:refnum<visa-resource-name>)  [unwired: 7 in]
          }
        }
      }
    }
    n69 = Unbundle By Name(w127) -> ("status"=w128:bool)
    n70 = Compound Arithmetic op=OR(w128, w124) -> (w126:bool)
  }
  n71 = Unbundle By Name(w44) -> ("Frequency"=w43:dbl)
  n72 = call-poly <vilib>:"DAQmx Trigger.vi"("task/channels in"=w93, "source"="Digital Trigger Source", "edge"="Edge", "error in"=w92) -> ("task out"=w52:refnum<k21>, "error out"=w51:errorcluster)  [unwired: 10 in]
  n73 = Divide(x="Sample Rate", y=w43) -> (x/y=w41:dbl)
  n74 = property class="DAQmx Trigger"(reference=w52, error in=w51, "Start.Retriggerable"=TRUE) -> (reference out=w3:refnum<k21>, error out=w2:errorcluster)
  n75 = Divide(x=w41, y=2.0) -> (x/y=w39:dbl)
  n76 = call-poly <vilib>:"DAQmx Create Virtual Channel.vi"("maximum value"="Max Voltage 2", "minimum value"="Min Voltage 2", "physical channels"="Physical Channel(s)", "error in"=w2) -> ("task out"=w76:refnum<k21>, "error out"=w77:errorcluster)  [unwired: 10 in]
  n77 = local read "Y-length"() -> (w29:dbl)
  n78 = local read "Step Y"() -> (w30:dbl)
  n79 = Obtain Queue(max queue size (-1, unlimited)=10000, name (unnamed)="data DAQ", element data type=dbl[] [] ("data")) -> (queue out=w35:refnum<queue>)  [unwired: 2 in, 2 out]
  n80 = Quotient & Remainder(x=w29, y=w30) -> (floor(x/y)=w28:dbl)  [unwired: 1 out]
  n81 = Initialize Array(0.0 ("element"), "Number of Samples 2") -> (w36:dbl[])
  n82 = Obtain Queue(max queue size (-1, unlimited)=10000, name (unnamed)="data Extraction", element data type=0.0) -> (queue out=w33:refnum<queue>)  [unwired: 2 in, 2 out]
  n83 = case shown="\"                    Test mode                   \"" "Tab Control 2" {
    tunnel: w3 -> [w259 w437]
    tunnel: [w273 w441] -> w82
    tunnel: [w272 w440] -> w81
    tunnel: w36 -> [w270 w439]
    tunnel: w2 -> [w258 w436]
    tunnel: w39 -> [w271 w438]
    tunnel: w35 -> [w269 _]
    tunnel: w33 -> [w268 _]
    tunnel: w28 -> [w262 _]
    frame "                          Scan mode                      ", Default {
      # "Column"
      # "Row"
      n84 = To Long Integer(number=w262) -> (32bit integer=w255:i32)
      n85 = disable-structure shown="Disabled" {
        frame Disabled {
          n86 = Decrement() -> (x-1=w279:dbl)  [unwired: 1 in]
          n87 = Decrement() -> (x-1=w278:dbl)  [unwired: 1 in]
          n88 = call "Surface_AxesScale.vi"("Y-axis Max"=w278, "X-axis max"=w279, "Auto Scale"=FALSE) -> ()  [unwired: 9 in]
        }
        frame Enabled {
        }
      }
      n89 = Increment(x=w255) -> (x+1=w254:i32)
      n90 = while {
        shift-right: [w339] -> _
        shift-left: w270 -> [w343]
        tunnel: w270 -> [w342]
        tunnel: w271 -> [w341]
        tunnel: w269 -> [w340]
        tunnel: w268 -> [w338]
        shift-right: [w322] -> w256
        shift-left: dbl[][] [] ("Out Array") -> [w337]
        shift-right: [w325] -> _
        shift-left: 0 -> [w336]
        shift-right: [w324] -> _
        shift-left: 0 -> [w331]
        shift-right: [w323] -> _
        shift-left: FALSE ("Output Direction") -> [w335]
        shift-right: [w326] -> _
        shift-left: 0.0 -> [w332]
        tunnel: w254 -> [w330]
        shift-right: [w320] -> _
        shift-left: FALSE -> [w321]
        shift-right: [w319] -> _
        shift-left: 0 -> [w318]
        stop <- w333 stop-if-true
        n91 = local read "Move X"() -> (w327:bool)
        n92 = local read "Scan"() -> (w328:bool)
        n93 = Equal?(x=w331, y=w330) -> (x = y?=w329:bool)
        n94 = And(x=w328, y=w327) -> (x .and. y?=w320:bool)
        n95 = case shown="True" w320 {
          selector: w320 -> [w348 w372]
          tunnel: w343 -> [w356 w377]
          tunnel: w342 -> [_ w389]
          tunnel: w341 -> [_ w388]
          tunnel: w340 -> [_ w387]
          tunnel: [w356 w386] -> w339
          tunnel: w338 -> [_ w385]
          tunnel: w337 -> [w353 w384]
          tunnel: [w351 w375] -> w322
          tunnel: w336 -> [w355 w383]
          tunnel: w331 -> [w346 w382]
          tunnel: w335 -> [w354 w369]
          tunnel: [w354 w381] -> w323
          tunnel: [w355 w380] -> w325
          tunnel: [w345 w379] -> w324
          tunnel: w318 -> [w344 w367]
          tunnel: [w350 w374] -> w326
          tunnel: w332 -> [w350 w373]
          tunnel: w321 -> [w349 w371]
          tunnel: [w344 w366] -> w319
          frame False {
            n96 = Not Equal?(x=w349, y=w348) -> (x != y?=w347:bool)
            n97 = case shown="True" w347 {
              tunnel: w346 -> [w357 w359]
              tunnel: [w357 w358] -> w345
              frame False {
              }
              frame True {
                n98 = Increment(x=w359) -> (x+1=w358:i32)
              }
            }
            n99 = call "CSV Open.vi"("2D Array In"=w353, "Open"="Open") -> ("2D Array Out"=w351:dbl[][])  [unwired: 9 in]
            n100 = case shown="True" "Open" {
              tunnel: w351 -> [_ w360]
              frame False {
              }
              frame True {
                n101 = Matrix Size(0:w360) -> (1:w361:i32, 2:w362:i32)
                n102 = Decrement(x=w361) -> (x-1=w365:i32)
                n103 = Decrement(x=w362) -> (x-1=w364:i32)
                n104 = call "Surface_AxesScale.vi"("Y-axis Max"=w364, "X-axis max"=w365, "Auto Scale"=FALSE) -> ()  [unwired: 9 in]
              }
            }
          }
          frame True {
            n105 = Not Equal?(x=w372, y=w371) -> (x != y?=w370:bool)
            n106 = local read "Average"() -> (w376:i32)
            n107 = case shown="True" w370 {
              tunnel: w369 -> [w393 w395]
              tunnel: [w393 w394] -> w368
              frame False {
              }
              frame True {
                n108 = Not(x=w395) -> (.not. x?=w394:bool)
              }
            }
            n109 = Increment(x=w367) -> (x+1=w366:i32)
            n110 = Dequeue Element(queue=w387) -> (element=w378:dbl[])  [unwired: 2 in, 3 out]
            n111 = Quotient & Remainder(x=w366, y=w376) -> (x-y*floor(x/y)=w390:i32)  [unwired: 1 out]
            n112 = Add(x=w378, y=w377) -> (x+y=w392:dbl[])
            n113 = Equal To 0?(x=w390) -> (x = 0?=w391:bool)
            n114 = case shown="True" w391 {
              tunnel: w376 -> [_ w417]
              tunnel: w392 -> [w401 w423]
              tunnel: [w401 w422] -> w386
              tunnel: w389 -> [_ w422]
              tunnel: w388 -> [_ w416]
              tunnel: w385 -> [_ w414]
              tunnel: w384 -> [w400 w409]
              tunnel: [w400 w410] -> w375
              tunnel: w383 -> [w399 w407]
              tunnel: w382 -> [w398 w406]
              tunnel: w368 -> [w397 w402]
              tunnel: [w397 w403] -> w381
              tunnel: [w399 w404] -> w380
              tunnel: [w398 w405] -> w379
              tunnel: [w396 w411] -> w374
              tunnel: w373 -> [w396 w408]
              frame False {
              }
              frame True {
                n115 = local read "Offset"() -> (w412:bool)
                n116 = Divide(x=w423, y=w417) -> (x/y=w413:dbl[])
                n117 = case shown="True" w412 {
                  tunnel: w416 -> [_ w432]
                  tunnel: w413 -> [w424 w426]
                  tunnel: [w424 w425] -> w415
                  frame False {
                  }
                  frame True {
                    w428 = 2.0 ("y")
                    n118 = Divide(x=w432, y=w428) -> (x/y=w433:dbl)
                    n119 = Index Array(array=w426, index #2=w433) -> (element #1=w430:dbl, element #2=w431:dbl)  [unwired: 1 in]
                    n120 = Add(x=w430, y=w431) -> (x+y=w429:dbl)
                    n121 = Divide(x=w429, y=w428) -> (x/y=w427:dbl)
                    n122 = Subtract(x=w426, y=w427) -> (x-y=w425:dbl[])
                  }
                }
                n123 = Array Subset(array=w415, length=w416) -> (w420:dbl[])  [unwired: 1 in]
                n124 = Array Subset(array=w415, index=w416, length=w416) -> (w419:dbl[])
                n125 = Subtract(x=w420, y=w419) -> (x-y=w418:dbl[])
                n126 = call "EletoMatr-no trigger.vi"("Input Array"=w409, "Input"=w408, "In Row"=w407, "In Column"=w406, "Input Direction"=w402) -> ("Out Array"=w410:dbl[][], "Output Direction"=w403:bool, "Out Row"=w404:i32, "Out Column"=w405:i32)  [unwired: 7 in]
                n127 = Add Array Elements(numeric array=w418) -> (sum=w421:dbl)
                n128 = Divide(x=w421, y=w416) -> (x/y=w411:dbl)
                "Feature Extraction 2" <- w411
                n129 = Lossy Enqueue Element(queue=w414, element=w411) -> ()  [unwired: 1 in, 4 out]
              }
            }
          }
        }
        n130 = local read "Stop Scan"() -> (w334:bool)
        n131 = Compound Arithmetic op=OR(w329, w334) -> (w333:bool)
        "숫자형 3" <- w336
        "Y line" <- w331
      }
      n132 = while {
        tunnel: w259 -> [w286]
        tunnel: [w293] -> w273
        tunnel: [w292] -> w272
        tunnel: w258 -> [w285]
        tunnel: w269 -> [w291]
        stop <- w290 stop-if-true
        n133 = And(x="Scan", y="Move X") -> (x .and. y?=w288:bool)
        n134 = case shown="True" w288 {
          tunnel: w286 -> [w295 w303]
          tunnel: [w295 w299] -> w293
          tunnel: [w294 w296] -> w292
          tunnel: w285 -> [w294 w302]
          tunnel: w291 -> [_ w304]
          frame False {
          }
          frame True {
            n135 = call <vilib>:"DAQmx Start Task.vi"("task/channels in"=w303, "error in"=w302) -> ("task out"=w301:refnum<k21>, "error out"=w300:errorcluster)  [unwired: 12 in]
            n136 = while {
              tunnel: w301 -> [w317]
              tunnel: [w316] -> w298
              tunnel: [w315] -> w297
              tunnel: w300 -> [w314]
              tunnel: w304 -> [w313]
              i -> [w305]
              stop <- w310 stop-if-true
              n137 = call-poly <vilib>:"DAQmx Read.vi"("task/channels in"=w317, "error in"=w314) -> ("task out"=w316:refnum<k21>, "data"=w306:dbl[], "error out"=w315:errorcluster)  [unwired: 11 in]
              n138 = Enqueue Element At Opposite End(queue=w313, element=w306) -> ()  [unwired: 2 in, 3 out]
              n139 = local read "Move X"() -> (w309:bool)
              n140 = local read "Scan"() -> (w308:bool)
              n141 = And(x=w308, y=w309) -> (x .and. y?=w307:bool)
              n142 = local read "Stop Scan"() -> (w311:bool)
              n143 = Unbundle By Name(w315) -> ("status"=w312:bool)
              n144 = Compound Arithmetic op=OR(w312, w311, invert w307) -> (w310:bool)
              "숫자형 2" <- w305
            }
            n145 = call <vilib>:"DAQmx Stop Task.vi"("task/channels in"=w298, "error in"=w297) -> ("task out"=w299:refnum<k21>, "error out"=w296:errorcluster)  [unwired: 12 in]
          }
        }
        n146 = local read "Stop Scan"() -> (w290:bool)
      }
      n147 = while {
        stop <- w282 stop-if-true
        n148 = Wait (ms)(milliseconds to wait=u32 100) -> ()  [unwired: 1 out]
        n149 = local read "3D Surface"() -> (w284:refnum<k7>)
        n150 = property class="CWGraph3D"(reference=w284, "ViewMode"="ViewMode Analysis") -> ()  [unwired: 1 in, 2 out]
        n151 = call <vilib>:"Basic Properties.vi"("3D graph"=w284, "plot style"="Plot style Analysis") -> ()  [unwired: 12 in, 2 out]
        n152 = local read "Stop Scan"() -> (w282:bool)
      }
      n153 = call <vilib>:"3D Surface.vi"("z matrix"=w256, "3D graph"="3D Surface") -> ()  [unwired: 8 in, 2 out]
      n154 = while {
        tunnel: w256 -> [w275]
        stop <- w274 stop-if-true
        n155 = call "CSV Save.vi"("Array"=w275, "Save Button"="Save Scan mode") -> ("Save Status"=w274:bool)  [unwired: 9 in]
      }
    }
    frame "                    Test mode                   " {
      n156 = call <vilib>:"DAQmx Start Task.vi"("task/channels in"=w437, "error in"=w436) -> ("task out"=w435:refnum<k21>, "error out"=w434:errorcluster)  [unwired: 12 in]
      n157 = while {
        tunnel: w435 -> [w463]
        tunnel: w434 -> [w462]
        tunnel: [w459] -> w440
        tunnel: [w460] -> w441
        shift-right: [w452] -> _
        shift-left: w439 -> [w454]
        tunnel: w439 -> [w450]
        shift-right: [w448] -> _
        shift-left: _ -> [w447]
        tunnel: w438 -> [w446]
        shift-right: [w445] -> _
        shift-left: _ -> [w444]
        i -> [w451]
        stop <- w461 stop-if-true
        n158 = Quotient & Remainder(x=w451, y="Average") -> (x-y*floor(x/y)=w457:i32)  [unwired: 1 out]
        n159 = call-poly <vilib>:"DAQmx Read.vi"("task/channels in"=w463, "error in"=w462) -> ("task out"=w460:refnum<k21>, "data"=w453:waveform(dbl), "error out"=w459:errorcluster)  [unwired: 11 in]
        n160 = Equal To 0?(x=w457) -> (x = 0?=w456:bool)
        n161 = Unbundle By Name(w453) -> ("Y"=w443:dbl[])
        n162 = Add(x=w443, y=w454) -> (x+y=w449:dbl[])
        n163 = case shown="True" w456 {
          tunnel: "Average" -> [_ w471]
          tunnel: w453 -> [_ w488]
          tunnel: w449 -> [w466 w487]
          tunnel: [w466 w486] -> w452
          tunnel: w450 -> [_ w486]
          tunnel: [w465 w482] -> w448
          tunnel: w447 -> [w465 w484]
          tunnel: w446 -> [_ w470]
          tunnel: [w464 w477] -> w445
          tunnel: w444 -> [w464 w479]
          frame False {
          }
          frame True {
            n164 = Divide(x=w487, y=w471) -> (x/y=w469:dbl[])
            n165 = case shown="True" "Offset" {
              tunnel: w470 -> [_ w497]
              tunnel: w469 -> [w489 w491]
              tunnel: [w489 w490] -> w467
              frame False {
              }
              frame True {
                w493 = 2.0 ("y")
                n166 = Divide(x=w497, y=w493) -> (x/y=w498:dbl)
                n167 = Index Array(array=w491, index #2=w498) -> (element #1=w495:dbl, element #2=w496:dbl)  [unwired: 1 in]
                n168 = Add(x=w495, y=w496) -> (x+y=w494:dbl)
                n169 = Divide(x=w494, y=w493) -> (x/y=w492:dbl)
                n170 = Subtract(x=w491, y=w492) -> (x-y=w490:dbl[])
              }
            }
            n171 = Bundle By Name(cluster=w488, "Y"=w467) -> (w476:waveform(dbl))
            n172 = Array Subset(array=w467, length=w470) -> (w475:dbl[])  [unwired: 1 in]
            n173 = Array Subset(array=w467, index=w470, length=w470) -> (w474:dbl[])
            n174 = Subtract(x=w475, y=w474) -> (x-y=w473:dbl[])
            n175 = xnode "Spectral Measurements"("신호"=w476) -> ("PSD"=w480:cluster{"f0":dbl, "df":dbl, "magnitude":dbl[]})  [unwired: 1 in, 1 out]
            n176 = Add Array Elements(numeric array=w473) -> (sum=w481:dbl)
            n177 = Divide(x=w481, y=w470) -> (x/y=→"Feature Extraction":dbl)
            n178 = case shown="True" "2 Plots" {
              tunnel: [w502 w508] -> w485
              tunnel: w484 -> [_ w507]
              tunnel: [w501 w507] -> w482
              tunnel: w476 -> [w501 w503]
              tunnel: w480 -> [w499 w505]
              tunnel: [w500 w506] -> w478
              tunnel: w479 -> [_ w504]
              tunnel: [w499 w504] -> w477
              frame False {
                n179 = Build Array(w499, w499) -> (w500:cluster{"f0":dbl, "df":dbl, "magnitude":dbl[]}[])
                n180 = Build Array(w501, w501) -> (w502:waveform(dbl)[])
              }
              frame True {
                n181 = Build Array(w504, w505) -> (w506:cluster{"f0":dbl, "df":dbl, "magnitude":dbl[]}[])
                n182 = Build Array(w507, w503) -> (w508:waveform(dbl)[])
              }
            }
            "Power spectral density" <- w478
            "Hall sensors signal" <- w485
          }
        }
        n183 = local read "Stop Scan"() -> (w442:bool)
        n184 = Unbundle By Name(w459) -> ("status"=w458:bool)
        n185 = Or(x=w458, y=w442) -> (x .or. y?=w461:bool)
      }
    }
  }
  n186 = call-poly <vilib>:"DAQmx Timing.vi"("task/channels in"=w76, "sample mode"=w78, "rate"="Sample Rate 2", "source"="Sample Clock Source", "error in"=w77) -> ("task out"=w80:refnum<k21>, "error out"=w79:errorcluster)  [unwired: 9 in]
  n187 = property class="DAQmx Timing"(reference=w80, error in=w79) -> (reference out=w62:refnum<k21>, error out=w66:errorcluster, "SampClk.Rate"=w64:dbl)
  "Actual Sample Rate 2" <- w64
  n188 = To Double Precision Float(number="Number of Samples") -> (double precision float=w59:dbl)
  n189 = call <vilib>:"Simple Error Handler.vi"("error in (no error)"=w25) -> ()  [unwired: 4 in, 5 out]
  n190 = Bundle By Name(cluster=cluster{"Fs":dbl, "#s":dbl} {"Fs"=1000.0, "#s"=1000.0} ("sampling info"), "#s"=w59, "Fs"=w64) -> (w63:cluster{"Fs":dbl, "#s":dbl})
  n191 = for {
    tunnel: w66 -> [w526]
    tunnel: w63 -> [w525]
    tunnel: [w524] -> w60
    tunnel: "Output Array" -> [w523] mode=indexing
    tunnel: [w520] -> w57 mode=indexing
    n192 = Unbundle By Name(w523) -> ("Waveform Type"=w522:u16, "Frequency"=w521:dbl, "Amplitude"=w518:dbl)
    n193 = call <vilib>:"Basic Function Generator.vi"("square wave duty cycle (%)"="Duty cycle %", "sampling info"=w525, "signal type"=w522, "error in (no error)"=w526, "amplitude"=w518, "frequency"=w521) -> ("error out"=w524:errorcluster, "signal out"=w520:waveform(dbl))  [unwired: 3 in, 1 out]
  }
  "Waveform Graph 2" <- w57
  n194 = call-poly <vilib>:"DAQmx Write.vi"("task/channels in"=w62, "data"=w57, "error in"=w60) -> ("task out"=w61:refnum<k21>, "error out"=w48:errorcluster)  [unwired: 10 in, 1 out]
  n195 = call <vilib>:"DAQmx Start Task.vi"("task/channels in"=w61, "error in"=w48) -> ("task out"=w75:refnum<k21>, "error out"=w49:errorcluster)  [unwired: 12 in]
  n196 = while {
    tunnel: w75 -> [w535]
    tunnel: w49 -> [w534]
    tunnel: [w532] -> w73
    tunnel: [w533] -> w74
    stop <- w527 stop-if-true
    n197 = call <vilib>:"DAQmx Is Task Done.vi"("task/channels in"=w535, "error in"=w534) -> ("task out"=w533:refnum<k21>, "error out"=w532:errorcluster)  [unwired: 11 in, 1 out]
    n198 = local read "Stop Scan"() -> (w530:bool)
    n199 = Unbundle By Name(w532) -> ("status"=w528:bool)
    n200 = Wait Until Next ms Multiple(millisecond multiple=u32 100) -> ()  [unwired: 1 out]
    n201 = Compound Arithmetic op=OR(w528, "Stop", w530) -> (w527:bool)
  }
  n202 = while {
    tunnel: w5 -> [w541]
    tunnel: [w539] -> _
    tunnel: w4 -> [w540]
    tunnel: [w538] -> _
    stop <- w537 stop-if-true
    n203 = local read "Scan"() -> (w536:bool)
    n204 = case shown="True" w536 {
      selector: w536 -> [_ w580]
      tunnel: [w543 w585] -> w539
      tunnel: w541 -> [w545 w582]
      tunnel: w540 -> [w544 w581]
      tunnel: [w542 w584] -> w538
      tunnel: [FALSE w587] -> w537
      frame False {
        n205 = while {
          tunnel: w544 -> [w554]
          tunnel: [w549] -> w543
          tunnel: [w548] -> w542
          tunnel: w545 -> [w547]
          stop <- w561 stop-if-true
          # "Stop at LS"
          # "Send command and get position"
          n206 = local read "Travel per Pulse (mm)"() -> (w557:dbl)
          n207 = local read "Cur. Pos X"() -> (w551:dbl)
          n208 = local read "Cur. Pos Y"() -> (w550:dbl)
          n209 = call "Sigma_GetPos.vi"("VISA resource name"=w547, "Travel per Pulse (mm)"=w557, "Init Pos X (mm)"=w551, "Init  Pos Y (mm)"=w550, "error in (no error)"=w554) -> ("Pos X (mm)"=w553:dbl, "Pos Y (mm)"=w552:dbl, "VISA resource name out"=w556:refnum<visa-resource-name>, "State String"=w558:string, "error out"=w555:errorcluster)  [unwired: 6 in]
          n210 = local write "Cur. Pos X"(w553) -> ()
          n211 = local write "Cur. Pos Y"(w552) -> ()
          n212 = Wait Until Next ms Multiple(millisecond multiple=u32 250) -> ()  [unwired: 1 out]
          n213 = case shown="\"K\", Default" w558 {
            tunnel: [w564 w569 w574 w579] -> w549
            tunnel: [w563 w568 w573 w578] -> w548
            tunnel: w556 -> [w564 w566 w571 w576]
            tunnel: w555 -> [w563 w565 w570 w575]
            frame "K", Default {
            }
            frame "L" {
              n214 = call "Sigma_Stop.vi"("Axis (1)"="1", "error in (no error)"=w565, "VISA resource name"=w566) -> ("error out"=w568:errorcluster, "VISA resource name out"=w569:refnum<visa-resource-name>)  [unwired: 7 in]
            }
            frame "M" {
              n215 = call "Sigma_Stop.vi"("Axis (1)"="2", "error in (no error)"=w570, "VISA resource name"=w571) -> ("error out"=w573:errorcluster, "VISA resource name out"=w574:refnum<visa-resource-name>)  [unwired: 7 in]
            }
            frame "W" {
              n216 = call "Sigma_Stop.vi"("Axis (1)"="W", "error in (no error)"=w575, "VISA resource name"=w576) -> ("error out"=w578:errorcluster, "VISA resource name out"=w579:refnum<visa-resource-name>)  [unwired: 7 in]
            }
          }
          n217 = Unbundle By Name(w548) -> ("status"=w562:bool)
          n218 = local read "Scan"() -> (w560:bool)
          n219 = Compound Arithmetic op=OR(w562, w560) -> (w561:bool)
        }
      }
      frame True {
        n220 = local read "Travel per Pulse (mm)"() -> (w583:dbl)
        n221 = local write "Move X"(w580) -> ()
        n222 = local read "Cur. Pos Y"() -> (w588:dbl)
        n223 = while {
          shift-right: [w608] -> _
          shift-left: TRUE ("Direction (+)") -> [w621]
          tunnel: w588 -> [w620]
          tunnel: [w616] -> w587
          tunnel: w582 -> [w623]
          tunnel: w581 -> [w622]
          tunnel: [w609] -> w585
          tunnel: [w606] -> w584
          tunnel: w583 -> [w597]
          stop <- w616 stop-if-true
          # "5. Stop scan condition"
          # "3. Run Step Y"
          # "2. wait until run to X-length"
          # "1. Move in X axis\n    Invert direction after moved Step Y"
          # "4. Update Y Possition"
          n224 = flat-sequence {
            tunnel: w623 -> [w629]
            tunnel: w622 -> [w628]
            tunnel: w621 -> [w634]
            tunnel: w620 -> [w632]
            tunnel: [w633] -> w596
            tunnel: [w627] -> w594
            tunnel: [w626] -> w592
            tunnel: [w632] -> w590
            tunnel: w597 -> [w625]
            tunnel: w596 -> [w639]
            tunnel: [w639] -> w595
            tunnel: w594 -> [w638]
            tunnel: [w638] -> w593
            tunnel: w592 -> [w637]
            tunnel: [w637] -> w591
            tunnel: w590 -> [w636]
            tunnel: [w636] -> w589
            tunnel: w595 -> [w642]
            tunnel: w593 -> [w647]
            tunnel: w591 -> [w646]
            tunnel: w589 -> [w643]
            tunnel: [w645] -> w615
            tunnel: [w644] -> w614
            tunnel: [w643] -> w610
            tunnel: [w642] -> w608
            tunnel: [w695] -> w605
            tunnel: w615 -> [w695]
            tunnel: [w694] -> w603
            tunnel: w614 -> [w694]
            tunnel: [w693] -> w601
            tunnel: w610 -> [w693]
            tunnel: w605 -> [w703]
            tunnel: [w703] -> w604
            tunnel: w603 -> [w702]
            tunnel: [w702] -> w602
            tunnel: w601 -> [w697]
            tunnel: [w698] -> w600
            tunnel: [w713] -> w619
            tunnel: [w712] -> w618
            tunnel: w604 -> [w709]
            tunnel: w602 -> [w708]
            tunnel: w600 -> [w705]
            tunnel: w619 -> [w727]
            tunnel: w618 -> [w726]
            tunnel: [w725] -> w611
            tunnel: [w724] -> w607
            tunnel: [w776] -> w613
            tunnel: [w775] -> w612
            tunnel: w611 -> [w775]
            tunnel: w607 -> [w776]
            tunnel: [w774] -> w598
            tunnel: w613 -> [w789]
            tunnel: [w790] -> w606
            tunnel: w612 -> [w790]
            tunnel: [w789] -> w609
            tunnel: [w788] -> w599
            tunnel: w598 -> [w788]
            frame #0 {
              n225 = local read "X-length"() -> (w631:dbl)
              n226 = local write "Move X"(FALSE ("Move X")) -> ()
              n227 = Not(x=w634) -> (.not. x?=w633:bool)
              n228 = call "Sigma_MoveAbs.vi"("Direction (+)"=w633, "Axis (1)"=1, "error in (no error)"=w628, "Travel (1mm)"=w631, "Travel per Pulse (0.004mm)"=w625, "VISA resource name"=w629) -> ("error out"=w626:errorcluster, "VISA resource name out"=w627:refnum<visa-resource-name>)  [unwired: 4 in]
            }
            frame #1 {
              n229 = Wait (ms)(milliseconds to wait=10.0 ("y")) -> ()  [unwired: 1 out]
            }
            frame #2 {
              n230 = local read "Cur. Pos X"() -> (w640:dbl)
              n231 = local read "Cur. Pos Y"() -> (w641:dbl)
              n232 = while {
                tunnel: w647 -> [w660]
                tunnel: w646 -> [w661]
                tunnel: [w659] -> w645
                tunnel: [w658] -> w644
                shift-right: [w652] -> _
                shift-left: w641 -> [w651]
                shift-right: [w653] -> _
                shift-left: w640 -> [w650]
                tunnel: w640 -> [w649]
                stop <- w668 stop-if-true
                # "Stop at LS"
                # "Send command and get position"
                n233 = local read "Travel per Pulse (mm)"() -> (w664:dbl)
                n234 = local read "X-length"() -> (w656:dbl)
                n235 = Wait Until Next ms Multiple(millisecond multiple=u32 100) -> ()  [unwired: 1 out]
                n236 = call "Sigma_GetPos.vi"("VISA resource name"=w660, "Travel per Pulse (mm)"=w664, "Init Pos X (mm)"=w650, "Init  Pos Y (mm)"=w651, "error in (no error)"=w661) -> ("Pos X (mm)"=w653:dbl, "Pos Y (mm)"=w652:dbl, "VISA resource name out"=w663:refnum<visa-resource-name>, "State String"=w665:string, "error out"=w662:errorcluster)  [unwired: 6 in]
                n237 = Subtract(x=w649, y=w653) -> (x-y=w655:dbl)
                n238 = local write "Cur. Pos X"(w653) -> ()
                n239 = local write "Cur. Pos Y"(w652) -> ()
                n240 = local write "Move X"(TRUE ("Move X")) -> ()
                n241 = Absolute Value(x=w655) -> (abs(x)=w657:dbl)
                n242 = Greater Or Equal?(x=w657, y=w656) -> (x >= y?=w654:bool)
                n243 = local read "Stop Scan"() -> (w667:bool)
                n244 = case shown="\"K\", Default" w665 {
                  tunnel: [w671 w676 w681 w686] -> w659
                  tunnel: [w670 w675 w680 w685] -> w658
                  tunnel: w663 -> [w671 w673 w678 w683]
                  tunnel: w662 -> [w670 w672 w677 w682]
                  frame "K", Default {
                  }
                  frame "L" {
                    n245 = call "Sigma_Stop.vi"("Axis (1)"="1", "error in (no error)"=w672, "VISA resource name"=w673) -> ("error out"=w675:errorcluster, "VISA resource name out"=w676:refnum<visa-resource-name>)  [unwired: 7 in]
                  }
                  frame "M" {
                    n246 = call "Sigma_Stop.vi"("Axis (1)"="2", "error in (no error)"=w677, "VISA resource name"=w678) -> ("error out"=w680:errorcluster, "VISA resource name out"=w681:refnum<visa-resource-name>)  [unwired: 7 in]
                  }
                  frame "W" {
                    n247 = call "Sigma_Stop.vi"("Axis (1)"="W", "error in (no error)"=w682, "VISA resource name"=w683) -> ("error out"=w685:errorcluster, "VISA resource name out"=w686:refnum<visa-resource-name>)  [unwired: 7 in]
                  }
                }
                n248 = Unbundle By Name(w658) -> ("status"=w669:bool)
                n249 = Compound Arithmetic op=OR(w669, w667, w654) -> (w668:bool)
              }
            }
            frame #3 {
              n250 = local read "1 Rate"() -> (w691:dbl)
              n251 = local read "Travel per Pulse (mm)"() -> (w692:dbl)
              n252 = local write "Move X"(FALSE ("Move X")) -> ()
              n253 = Divide(x=w691, y=w692) -> (x/y=w688:dbl)
              n254 = Add(x=w688, y=100.0) -> (x+y=w690:dbl)
              n255 = Wait (ms)(milliseconds to wait=w690) -> ()  [unwired: 1 out]
            }
            frame #4 {
              n256 = local read "Y-length"() -> (w696:dbl)
              n257 = local read "Cur. Pos Y"() -> (w701:dbl)
              n258 = Subtract(x=w701, y=w697) -> (x-y=w700:dbl)
              n259 = Absolute Value(x=w700) -> (abs(x)=w699:dbl)
              n260 = Greater Or Equal?(x=w699, y=w696) -> (x >= y?=w698:bool)
            }
            frame #5 {
              # "Stop Y"
              n261 = local read "Step Y"() -> (w711:dbl)
              n262 = local read "Y-length"() -> (w710:dbl)
              n263 = local read "Stop Scan"() -> (w707:bool)
              n264 = Greater Or Equal?(x=w711, y=w710) -> (x >= y?=w706:bool)
              n265 = Compound Arithmetic op=OR(w705, w706, w707) -> (w704:bool)
              n266 = case shown="False" w704 {
                tunnel: [w718 w723] -> w713
                tunnel: [w717 w722] -> w712
                tunnel: w709 -> [w715 w723]
                tunnel: w708 -> [w714 w722]
                frame False {
                  n267 = local read "Travel per Pulse (mm)"() -> (w716:dbl)
                  n268 = local read "Step Y"() -> (w720:dbl)
                  n269 = call "Sigma_MoveAbs.vi"("Axis (1)"=2, "error in (no error)"=w714, "Travel (1mm)"=w720, "Travel per Pulse (0.004mm)"=w716, "VISA resource name"=w715) -> ("error out"=w717:errorcluster, "VISA resource name out"=w718:refnum<visa-resource-name>)  [unwired: 5 in]
                }
                frame True {
                  n270 = local write "Stop Scan"(TRUE ("Stop Scan")) -> ()
                }
              }
            }
            frame #6 {
              n271 = disable-structure shown="Disabled" {
                disable-tunnel: w727 -> [w733 w773]
                disable-tunnel: w726 -> [w732 w772]
                disable-tunnel: [w731 w772] -> w725
                disable-tunnel: [w730 w773] -> w724
                frame Disabled {
                  n272 = local read item#-1() -> (w729)
                  n273 = local read item#-1() -> (w728)
                  n274 = while {
                    tunnel: w733 -> [w745]
                    tunnel: w732 -> [w746]
                    tunnel: [w744] -> w730
                    tunnel: [w743] -> w731
                    shift-right: [w738] -> _
                    shift-left: w728 -> [w735]
                    shift-right: [w737] -> _
                    shift-left: w729 -> [w736]
                    tunnel: w728 -> [w734]
                    stop <- w753 stop-if-true
                    # "Stop at LS"
                    # "Send command and get position"
                    n275 = local read item#-1() -> (w749)
                    n276 = Wait Until Next ms Multiple(millisecond multiple=u32 100) -> ()  [unwired: 1 out]
                    n277 = local read item#-1() -> (w741)
                    n278 = call "Sigma_GetPos.vi"("VISA resource name"=w745, "Travel per Pulse (mm)"=w749, "Init Pos X (mm)"=w736, "Init  Pos Y (mm)"=w735, "error in (no error)"=w746) -> ("Pos X (mm)"=w737:dbl, "Pos Y (mm)"=w738:dbl, "VISA resource name out"=w748:refnum<visa-resource-name>, "State String"=w750:string, "error out"=w747:errorcluster)  [unwired: 6 in]
                    n279 = Subtract(x=w734, y=w738) -> (x-y=w740:dbl)
                    n280 = local write item#-1(w737) -> ()
                    n281 = local write item#-1(w738) -> ()
                    n282 = Absolute Value(x=w740) -> (abs(x)=w742:dbl)
                    n283 = Greater Or Equal?(x=w742, y=w741) -> (x >= y?=w739:bool)
                    n284 = local read "Stop Scan 2"() -> (w752:bool)
                    n285 = case shown="\"K\", Default" w750 {
                      tunnel: [w756 w761 w766 w771] -> w744
                      tunnel: [w755 w760 w765 w770] -> w743
                      tunnel: w748 -> [w756 w758 w763 w768]
                      tunnel: w747 -> [w755 w757 w762 w767]
                      frame "K", Default {
                      }
                      frame "L" {
                        n286 = call "Sigma_Stop.vi"("Axis (1)"="1", "error in (no error)"=w757, "VISA resource name"=w758) -> ("error out"=w760:errorcluster, "VISA resource name out"=w761:refnum<visa-resource-name>)  [unwired: 7 in]
                      }
                      frame "M" {
                        n287 = call "Sigma_Stop.vi"("Axis (1)"="2", "error in (no error)"=w762, "VISA resource name"=w763) -> ("error out"=w765:errorcluster, "VISA resource name out"=w766:refnum<visa-resource-name>)  [unwired: 7 in]
                      }
                      frame "W" {
                        n288 = call "Sigma_Stop.vi"("Axis (1)"="W", "error in (no error)"=w767, "VISA resource name"=w768) -> ("error out"=w770:errorcluster, "VISA resource name out"=w771:refnum<visa-resource-name>)  [unwired: 7 in]
                      }
                    }
                    n289 = Unbundle By Name(w743) -> ("status"=w754:bool)
                    n290 = Compound Arithmetic op=OR(w754, w752, w739) -> (w753:bool)
                  }
                }
                frame Enabled {
                }
              }
            }
            frame #7 {
              n291 = local read "Stop Scan"() -> (w774:bool)
            }
            frame #8 {
              # "waiting for stop speed\naxis 2 + 100ms more"
              n292 = local read "2 Rate"() -> (w780:dbl)
              n293 = local read "2 Max"() -> (w786:dbl)
              n294 = local read "Travel per Pulse (mm)"() -> (w779:dbl)
              n295 = local read "Step Y"() -> (w787:dbl)
              n296 = Compound Arithmetic op=MULTIPLY(w780, invert w779, 2.0 ("value")) -> (w777:dbl)
              n297 = Compound Arithmetic op=MULTIPLY(w787, invert w786, 1000.0 ("value")) -> (w784:dbl)
              n298 = Add(x=w777, y=w784) -> (x+y=w783:dbl)
              n299 = Add(x=w783, y=100.0) -> (x+y=w781:dbl)
              n300 = Wait (ms)(milliseconds to wait=w781) -> ()  [unwired: 1 out]
            }
          }
          n301 = Unbundle By Name(w606) -> ("status"=w617:bool)
          n302 = Compound Arithmetic op=OR(w617, w599) -> (w616:bool)
        }
      }
    }
  }
  n303 = call <vilib>:"DAQmx Clear Task.vi"("task in"=w74, "error in"=w73) -> ("error out"=w72:errorcluster)  [unwired: 13 in]
  n304 = call <vilib>:"Simple Error Handler.vi"("error in (no error)"=w72) -> ()  [unwired: 4 in, 5 out]
  n305 = call <vilib>:"DAQmx Clear Task.vi"("task in"=w82, "error in"=w81) -> ("error out"=w91:errorcluster)  [unwired: 13 in]
  n306 = call <vilib>:"Simple Error Handler.vi"("error in (no error)"=w91) -> ()  [unwired: 4 in, 5 out]
  n307 = call <vilib>:"Simple Error Handler.vi"() -> ()  [unwired: 5 in, 5 out]
